vi "七段数码管788.vi"() -> ()   [LabVIEW 2025]
uses:
  <vilib>/Instr/_visa.llb/VISA Configure Serial Port (Instr).vi
panel:
  out "Number of Bytes":u32
  in  "?":bool
  in  "?":bool
  in  "?":bool
  in  "停止":bool
  out "比赛次数个位":T1={"1"=TRUE, "2"=TRUE, "3"=TRUE, "4"=TRUE, "5"=TRUE, "6"=TRUE, "7"=FALSE}
  out "比赛次数十位":T1={"1"=TRUE, "2"=TRUE, "3"=TRUE, "4"=TRUE, "5"=TRUE, "6"=TRUE, "7"=FALSE}
  out "读取缓冲区 5":string
  in  "VISA resource":refnum<visa-resource-name> caption="VISA资源名称"
  out "7 3":bool
  out "6 3":bool
  out "5 3":bool
  out "4 3":bool
  out "3 3":bool
  out "2 3":bool
  out "1 3":bool
  out "7 2":bool
  out "6 2":bool
  out "5 2":bool
  out "4 2":bool
  out "3 2":bool
  out "2 2":bool
  out "1 2":bool
  out "7":bool
  out "6":bool
  out "5":bool
  out "4":bool
  out "3":bool
  out "2":bool
  out "1":bool
  out "结束":bool
  out "计时":bool=TRUE
  out "候场/暂停":bool
  in  "比赛状态":bool
  out "指示灯1 2":bool=TRUE
  out "指示灯2 2":bool=TRUE
  out "蓝方本局得分个位":T1={"1"=TRUE, "2"=TRUE, "3"=TRUE, "4"=TRUE, "5"=TRUE, "6"=TRUE, "7"=FALSE}
  out "蓝方本局得分十位":T1={"1"=TRUE, "2"=TRUE, "3"=TRUE, "4"=TRUE, "5"=TRUE, "6"=TRUE, "7"=FALSE}
  out "红方本局得分个位":T1={"1"=TRUE, "2"=TRUE, "3"=TRUE, "4"=TRUE, "5"=TRUE, "6"=TRUE, "7"=FALSE}
  out "红方本局得分十位":T1={"1"=TRUE, "2"=TRUE, "3"=TRUE, "4"=TRUE, "5"=TRUE, "6"=TRUE, "7"=FALSE}
  out "指示灯2":bool=TRUE
  out "指示灯1":bool=TRUE
  out "蓝方胜场得分个位":T1={"1"=TRUE, "2"=TRUE, "3"=TRUE, "4"=TRUE, "5"=TRUE, "6"=TRUE, "7"=FALSE}
  out "蓝方胜场比分十位":T1={"1"=TRUE, "2"=TRUE, "3"=TRUE, "4"=TRUE, "5"=TRUE, "6"=TRUE, "7"=FALSE}
  out "红方胜场比分个位":T1={"1"=TRUE, "2"=TRUE, "3"=TRUE, "4"=TRUE, "5"=TRUE, "6"=TRUE, "7"=FALSE}
  out "红方胜场比分十位":T1={"1"=TRUE, "2"=TRUE, "3"=TRUE, "4"=TRUE, "5"=TRUE, "6"=TRUE, "7"=FALSE}
  # "竹节人大作战数字擂台"
  # "比赛场次"
  # "比赛倒计时"
  # "红方"
  # "蓝方"
  # "本局得分"
  # "串口配置与操作区"
  # "胜场大比分"
  # "比赛状态"
  # "候场/暂停"
  # "计时"
  # "结束"
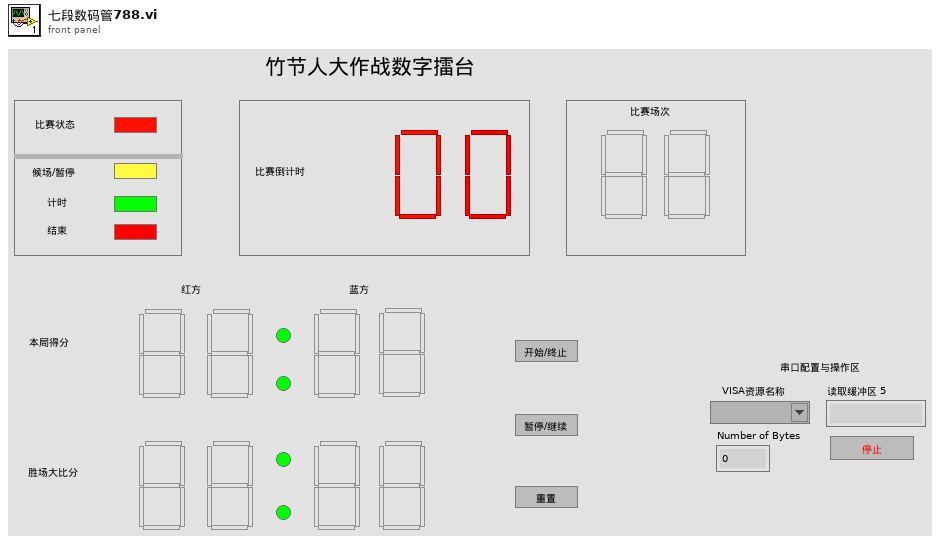
[diagram p1: front panel]
types:
  T1 = cluster{"1":bool, "2":bool, "3":bool, "4":bool, "5":bool, "6":bool, "7":bool}
  T2 = cluster{"7":bool, "6":bool, "5":bool, "4":bool, "3":bool, "2":bool, "1":bool}
  T3 = enum16{"big-endian, network order", "native, host order", "little-endian"}
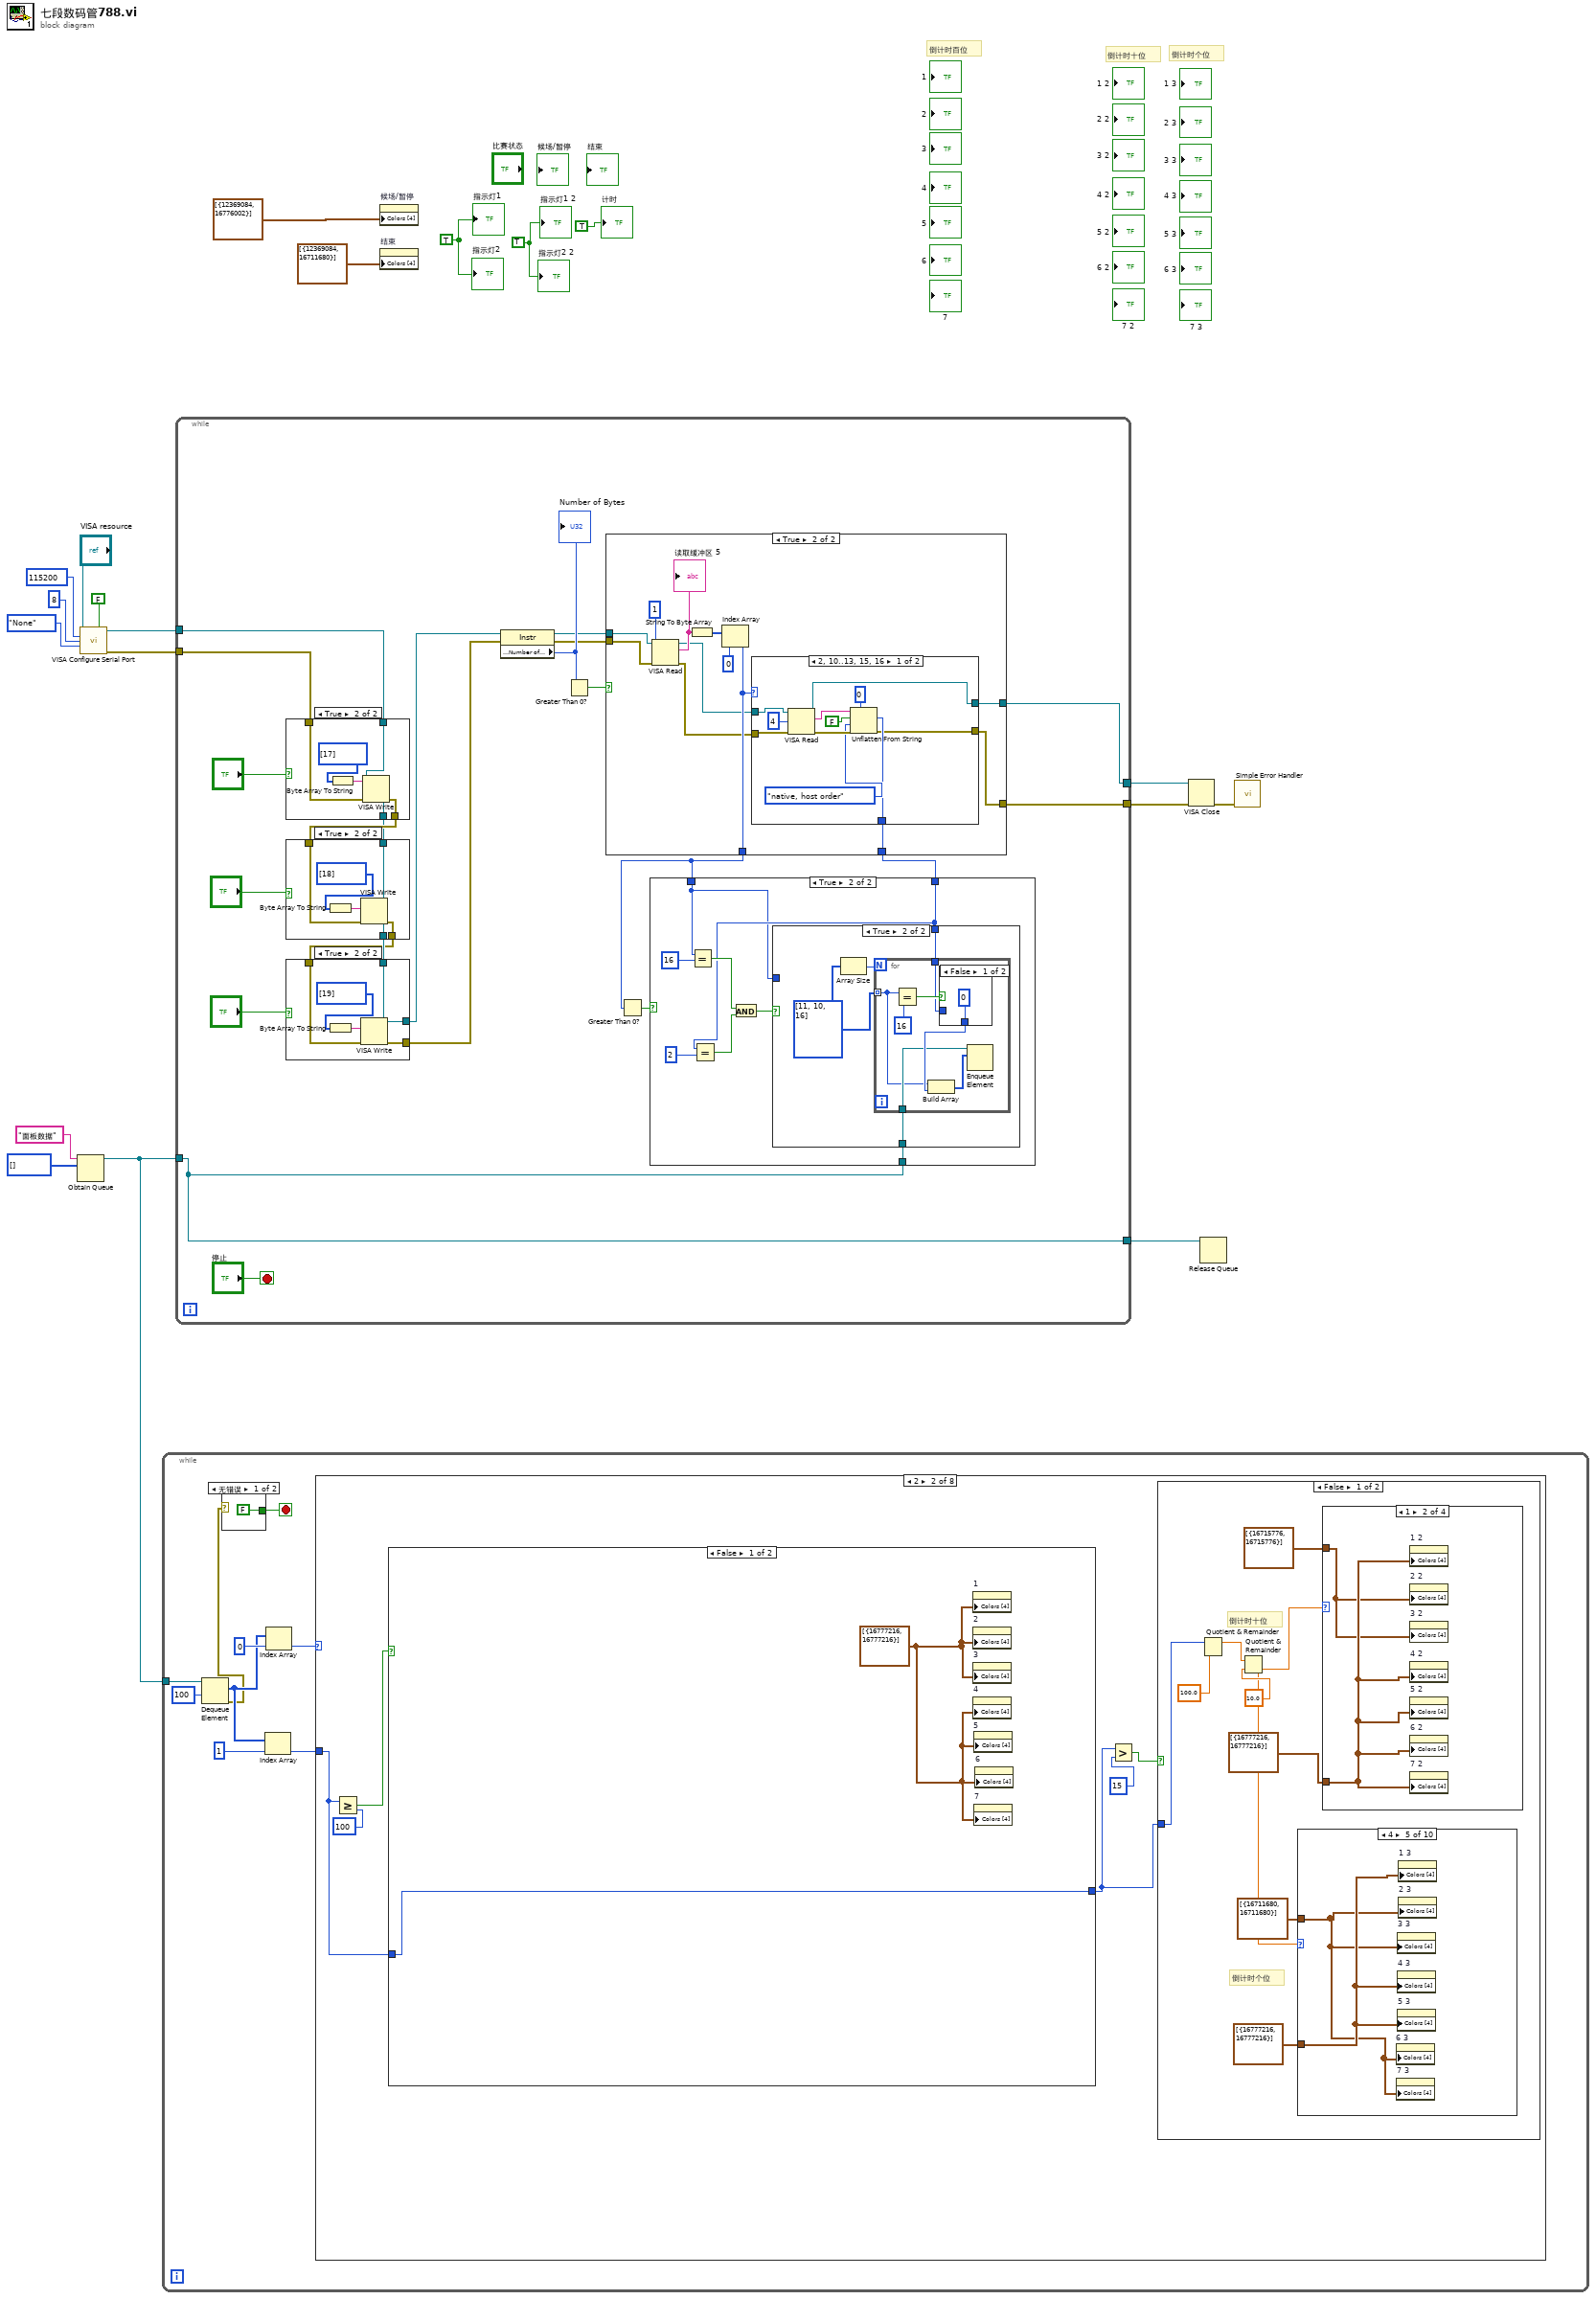
[diagram p0: block diagram]
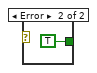
[diagram p2: hidden frame]
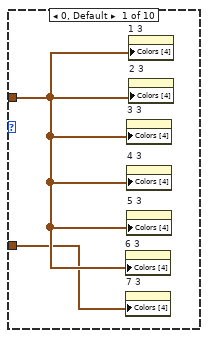
[diagram p4: hidden frame]
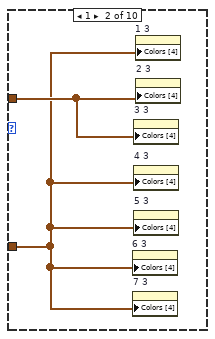
[diagram p5: hidden frame]
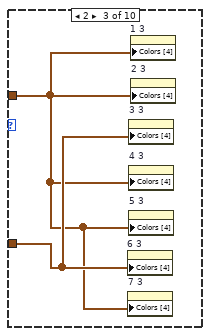
[diagram p6: hidden frame]
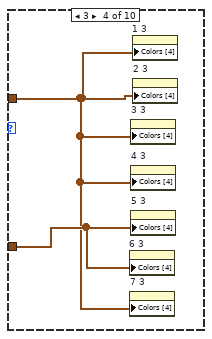
[diagram p7: hidden frame]
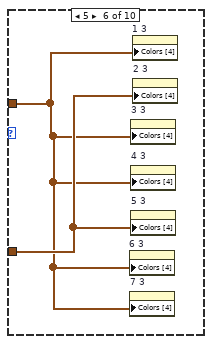
[diagram p8: hidden frame]
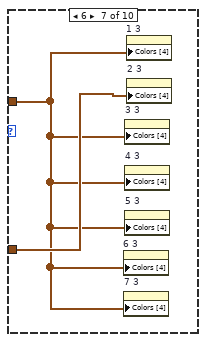
[diagram p9: hidden frame]
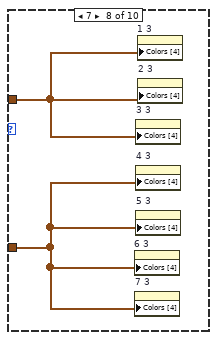
[diagram p10: hidden frame]
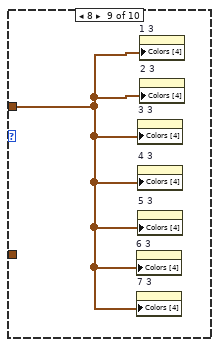
[diagram p11: hidden frame]
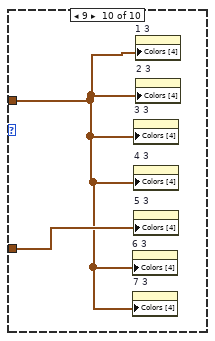
[diagram p12: hidden frame]
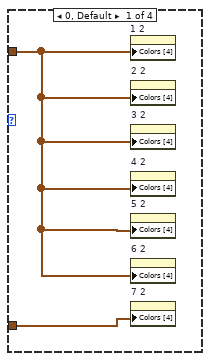
[diagram p13: hidden frame]
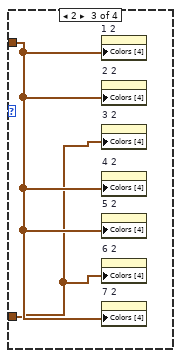
[diagram p14: hidden frame]
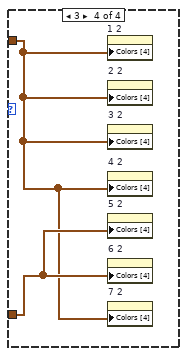
[diagram p15: hidden frame]
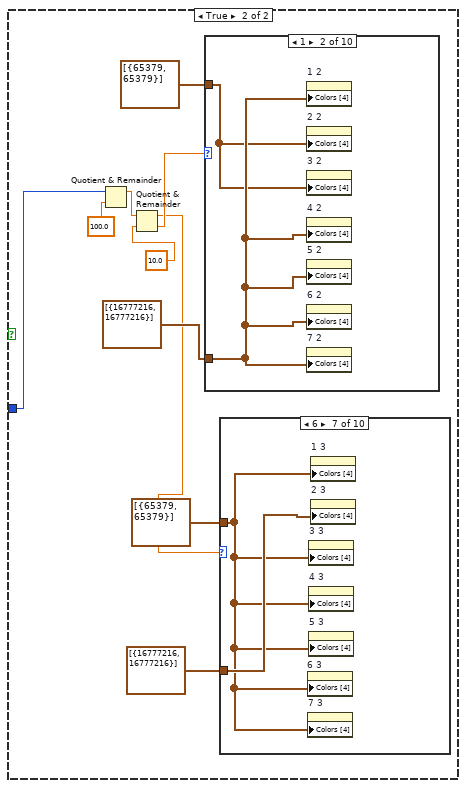
[diagram p16: hidden frame]
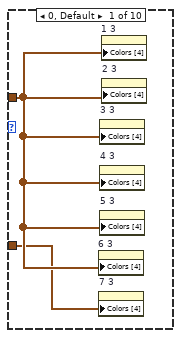
[diagram p17: hidden frame]
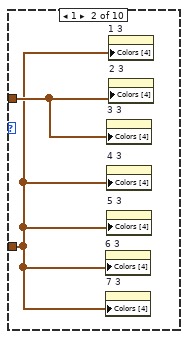
[diagram p18: hidden frame]
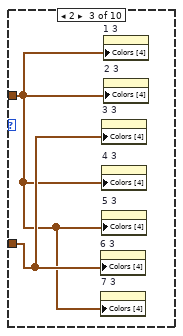
[diagram p19: hidden frame]
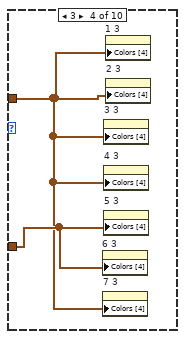
[diagram p20: hidden frame]
diagram:
  w15 = TRUE
  w16 = TRUE
  # "倒计时个位"
  # "倒计时十位"
  # "倒计时百位"
  n1 = Obtain Queue(name (unnamed)="面板数据" ("名称（未命名）"), element data type=i32[] []) -> (queue out=w2:refnum<queue>)  [unwired: 3 in, 2 out]
  n2 = call-poly "VISA Configure Serial Port"("VISA resource name"="VISA resource", "Enable Termination\nChar (T)"=FALSE ("Enable Termination\nChar (T)"), "baud rate (9600)"=u32 115200, "data bits (8)"=u16 8, "parity (0:none)"=enum16{"None", "Odd", "Even", "Mark", "Space"}."None") -> ("VISA resource name out"=w6:refnum<visa-resource-name>, "error out"=w5:errorcluster)  [unwired: 9 in]
  n3 = while {
    tunnel: w2 -> [w23]
    stop <- w24 stop-if-true
    n4 = Dequeue Element(queue=w23, timeout in ms (-1)=100 ("超时毫秒(-1)")) -> (element=w22:i32[], error out=w21:errorcluster)  [unwired: 1 in, 2 out]
    n5 = case shown="无错误" w21 {
      tunnel: [FALSE TRUE] -> w24
      frame No Error {
      }
      frame Error {
      }
    }
    n6 = Index Array(array=w22, index=1 ("索引")) -> (element=w25:i32)
    n7 = Index Array(array=w22, index=0 ("索引")) -> (element=w26:i32)
    n8 = case shown="2" w26 {
      tunnel: w25 -> [_ w33 w190 w219 w246 w271 w297 w321]
      frame Default {
      }
      frame 2 {
        n9 = Greater Or Equal?(x=w33, y=100) -> (x >= y?=w32:bool)
        n10 = case shown="False" w32 {
          tunnel: w33 -> [w123 w124]
          tunnel: [w123 w124] -> w31
          frame False {
            w122 = cluster{u32, u32}[] [{16777216, 16777216}] ("颜色[4]")
            n11 = property on="1" class="Bool (严格)"("Colors [4]"=w122) -> ()  [unwired: 2 in, 2 out]
            n12 = property on="2" class="Bool (严格)"("Colors [4]"=w122) -> ()  [unwired: 2 in, 2 out]
            n13 = property on="3" class="Bool (严格)"("Colors [4]"=w122) -> ()  [unwired: 2 in, 2 out]
            n14 = property on="4" class="Bool (严格)"("Colors [4]"=w122) -> ()  [unwired: 2 in, 2 out]
            n15 = property on="5" class="Bool (严格)"("Colors [4]"=w122) -> ()  [unwired: 2 in, 2 out]
            n16 = property on="7" class="Bool (严格)"("Colors [4]"=w122) -> ()  [unwired: 2 in, 2 out]
            n17 = property on="6" class="Bool (严格)"("Colors [4]"=w122) -> ()  [unwired: 2 in, 2 out]
          }
          frame True {
            w125 = cluster{u32, u32}[] [{16777216, 16777216}] ("颜色[4]")
            w126 = cluster{u32, u32}[] [{65379, 65379}] ("颜色[4]")
            n18 = Quotient & Remainder(x=w124, y=100.0) -> (x-y*floor(x/y)=w132:dbl, floor(x/y)=w128:dbl)
            n19 = Quotient & Remainder(x=w132, y=10.0) -> (x-y*floor(x/y)=w130:dbl, floor(x/y)=w131:dbl)
            n20 = case shown="0, 默认" w128 {
              tunnel: w126 -> [w172 w174 w176 w178 w180 w182 w184 w186 w187 w189]
              tunnel: w125 -> [w171 w173 w175 w177 w179 w181 w183 w185 _ w188]
              frame 0, Default {
                n21 = property on="1" class="Bool (严格)"("Colors [4]"=w172) -> ()  [unwired: 2 in, 2 out]
                n22 = property on="2" class="Bool (严格)"("Colors [4]"=w172) -> ()  [unwired: 2 in, 2 out]
                n23 = property on="5" class="Bool (严格)"("Colors [4]"=w172) -> ()  [unwired: 2 in, 2 out]
                n24 = property on="3" class="Bool (严格)"("Colors [4]"=w172) -> ()  [unwired: 2 in, 2 out]
                n25 = property on="4" class="Bool (严格)"("Colors [4]"=w172) -> ()  [unwired: 2 in, 2 out]
                n26 = property on="7" class="Bool (严格)"("Colors [4]"=w171) -> ()  [unwired: 2 in, 2 out]
                n27 = property on="6" class="Bool (严格)"("Colors [4]"=w172) -> ()  [unwired: 2 in, 2 out]
              }
              frame 1 {
                n28 = property on="1" class="Bool (严格)"("Colors [4]"=w173) -> ()  [unwired: 2 in, 2 out]
                n29 = property on="2" class="Bool (严格)"("Colors [4]"=w174) -> ()  [unwired: 2 in, 2 out]
                n30 = property on="5" class="Bool (严格)"("Colors [4]"=w173) -> ()  [unwired: 2 in, 2 out]
                n31 = property on="3" class="Bool (严格)"("Colors [4]"=w174) -> ()  [unwired: 2 in, 2 out]
                n32 = property on="4" class="Bool (严格)"("Colors [4]"=w173) -> ()  [unwired: 2 in, 2 out]
                n33 = property on="7" class="Bool (严格)"("Colors [4]"=w173) -> ()  [unwired: 2 in, 2 out]
                n34 = property on="6" class="Bool (严格)"("Colors [4]"=w173) -> ()  [unwired: 2 in, 2 out]
              }
              frame 2 {
                n35 = property on="1" class="Bool (严格)"("Colors [4]"=w176) -> ()  [unwired: 2 in, 2 out]
                n36 = property on="2" class="Bool (严格)"("Colors [4]"=w176) -> ()  [unwired: 2 in, 2 out]
                n37 = property on="3" class="Bool (严格)"("Colors [4]"=w175) -> ()  [unwired: 2 in, 2 out]
                n38 = property on="4" class="Bool (严格)"("Colors [4]"=w176) -> ()  [unwired: 2 in, 2 out]
                n39 = property on="5" class="Bool (严格)"("Colors [4]"=w176) -> ()  [unwired: 2 in, 2 out]
                n40 = property on="7" class="Bool (严格)"("Colors [4]"=w176) -> ()  [unwired: 2 in, 2 out]
                n41 = property on="6" class="Bool (严格)"("Colors [4]"=w175) -> ()  [unwired: 2 in, 2 out]
              }
              frame 3 {
                n42 = property on="1" class="Bool (严格)"("Colors [4]"=w178) -> ()  [unwired: 2 in, 2 out]
                n43 = property on="2" class="Bool (严格)"("Colors [4]"=w178) -> ()  [unwired: 2 in, 2 out]
                n44 = property on="3" class="Bool (严格)"("Colors [4]"=w178) -> ()  [unwired: 2 in, 2 out]
                n45 = property on="4" class="Bool (严格)"("Colors [4]"=w178) -> ()  [unwired: 2 in, 2 out]
                n46 = property on="5" class="Bool (严格)"("Colors [4]"=w177) -> ()  [unwired: 2 in, 2 out]
                n47 = property on="7" class="Bool (严格)"("Colors [4]"=w178) -> ()  [unwired: 2 in, 2 out]
                n48 = property on="6" class="Bool (严格)"("Colors [4]"=w177) -> ()  [unwired: 2 in, 2 out]
              }
              frame 4 {
                n49 = property on="1" class="Bool (严格)"("Colors [4]"=w179) -> ()  [unwired: 2 in, 2 out]
                n50 = property on="2" class="Bool (严格)"("Colors [4]"=w180) -> ()  [unwired: 2 in, 2 out]
                n51 = property on="3" class="Bool (严格)"("Colors [4]"=w180) -> ()  [unwired: 2 in, 2 out]
                n52 = property on="4" class="Bool (严格)"("Colors [4]"=w179) -> ()  [unwired: 2 in, 2 out]
                n53 = property on="5" class="Bool (严格)"("Colors [4]"=w179) -> ()  [unwired: 2 in, 2 out]
                n54 = property on="7" class="Bool (严格)"("Colors [4]"=w180) -> ()  [unwired: 2 in, 2 out]
                n55 = property on="6" class="Bool (严格)"("Colors [4]"=w180) -> ()  [unwired: 2 in, 2 out]
              }
              frame 5 {
                n56 = property on="1" class="Bool (严格)"("Colors [4]"=w182) -> ()  [unwired: 2 in, 2 out]
                n57 = property on="2" class="Bool (严格)"("Colors [4]"=w181) -> ()  [unwired: 2 in, 2 out]
                n58 = property on="3" class="Bool (严格)"("Colors [4]"=w182) -> ()  [unwired: 2 in, 2 out]
                n59 = property on="4" class="Bool (严格)"("Colors [4]"=w182) -> ()  [unwired: 2 in, 2 out]
                n60 = property on="5" class="Bool (严格)"("Colors [4]"=w181) -> ()  [unwired: 2 in, 2 out]
                n61 = property on="7" class="Bool (严格)"("Colors [4]"=w182) -> ()  [unwired: 2 in, 2 out]
                n62 = property on="6" class="Bool (严格)"("Colors [4]"=w182) -> ()  [unwired: 2 in, 2 out]
              }
              frame 6 {
                n63 = property on="1" class="Bool (严格)"("Colors [4]"=w184) -> ()  [unwired: 2 in, 2 out]
                n64 = property on="2" class="Bool (严格)"("Colors [4]"=w183) -> ()  [unwired: 2 in, 2 out]
                n65 = property on="3" class="Bool (严格)"("Colors [4]"=w184) -> ()  [unwired: 2 in, 2 out]
                n66 = property on="4" class="Bool (严格)"("Colors [4]"=w184) -> ()  [unwired: 2 in, 2 out]
                n67 = property on="5" class="Bool (严格)"("Colors [4]"=w184) -> ()  [unwired: 2 in, 2 out]
                n68 = property on="7" class="Bool (严格)"("Colors [4]"=w184) -> ()  [unwired: 2 in, 2 out]
                n69 = property on="6" class="Bool (严格)"("Colors [4]"=w184) -> ()  [unwired: 2 in, 2 out]
              }
              frame 7 {
                n70 = property on="1" class="Bool (严格)"("Colors [4]"=w186) -> ()  [unwired: 2 in, 2 out]
                n71 = property on="2" class="Bool (严格)"("Colors [4]"=w186) -> ()  [unwired: 2 in, 2 out]
                n72 = property on="3" class="Bool (严格)"("Colors [4]"=w186) -> ()  [unwired: 2 in, 2 out]
                n73 = property on="4" class="Bool (严格)"("Colors [4]"=w185) -> ()  [unwired: 2 in, 2 out]
                n74 = property on="5" class="Bool (严格)"("Colors [4]"=w185) -> ()  [unwired: 2 in, 2 out]
                n75 = property on="7" class="Bool (严格)"("Colors [4]"=w185) -> ()  [unwired: 2 in, 2 out]
                n76 = property on="6" class="Bool (严格)"("Colors [4]"=w185) -> ()  [unwired: 2 in, 2 out]
              }
              frame 8 {
                n77 = property on="1" class="Bool (严格)"("Colors [4]"=w187) -> ()  [unwired: 2 in, 2 out]
                n78 = property on="2" class="Bool (严格)"("Colors [4]"=w187) -> ()  [unwired: 2 in, 2 out]
                n79 = property on="3" class="Bool (严格)"("Colors [4]"=w187) -> ()  [unwired: 2 in, 2 out]
                n80 = property on="4" class="Bool (严格)"("Colors [4]"=w187) -> ()  [unwired: 2 in, 2 out]
                n81 = property on="5" class="Bool (严格)"("Colors [4]"=w187) -> ()  [unwired: 2 in, 2 out]
                n82 = property on="7" class="Bool (严格)"("Colors [4]"=w187) -> ()  [unwired: 2 in, 2 out]
                n83 = property on="6" class="Bool (严格)"("Colors [4]"=w187) -> ()  [unwired: 2 in, 2 out]
              }
              frame 9 {
                n84 = property on="1" class="Bool (严格)"("Colors [4]"=w189) -> ()  [unwired: 2 in, 2 out]
                n85 = property on="2" class="Bool (严格)"("Colors [4]"=w189) -> ()  [unwired: 2 in, 2 out]
                n86 = property on="3" class="Bool (严格)"("Colors [4]"=w189) -> ()  [unwired: 2 in, 2 out]
                n87 = property on="4" class="Bool (严格)"("Colors [4]"=w189) -> ()  [unwired: 2 in, 2 out]
                n88 = property on="5" class="Bool (严格)"("Colors [4]"=w188) -> ()  [unwired: 2 in, 2 out]
                n89 = property on="7" class="Bool (严格)"("Colors [4]"=w189) -> ()  [unwired: 2 in, 2 out]
                n90 = property on="6" class="Bool (严格)"("Colors [4]"=w189) -> ()  [unwired: 2 in, 2 out]
              }
            }
            n91 = case shown="0, 默认" w130 {
              tunnel: w126 -> [w134 w136 w137 w139 w141 w143 w145 w148 w149 w150]
              tunnel: w125 -> [w133 w135 w138 w140 w142 w144 w146 w147 _ w151]
              frame 0, Default {
                n92 = property on="6 3" class="Bool (严格)"("Colors [4]"=w134) -> ()  [unwired: 2 in, 2 out]
                n93 = property on="7 3" class="Bool (严格)"("Colors [4]"=w133) -> ()  [unwired: 2 in, 2 out]
                n94 = property on="3 3" class="Bool (严格)"("Colors [4]"=w134) -> ()  [unwired: 2 in, 2 out]
                n95 = property on="4 3" class="Bool (严格)"("Colors [4]"=w134) -> ()  [unwired: 2 in, 2 out]
                n96 = property on="5 3" class="Bool (严格)"("Colors [4]"=w134) -> ()  [unwired: 2 in, 2 out]
                n97 = property on="1 3" class="Bool (严格)"("Colors [4]"=w134) -> ()  [unwired: 2 in, 2 out]
                n98 = property on="2 3" class="Bool (严格)"("Colors [4]"=w134) -> ()  [unwired: 2 in, 2 out]
              }
              frame 1 {
                n99 = property on="6 3" class="Bool (严格)"("Colors [4]"=w135) -> ()  [unwired: 2 in, 2 out]
                n100 = property on="7 3" class="Bool (严格)"("Colors [4]"=w135) -> ()  [unwired: 2 in, 2 out]
                n101 = property on="3 3" class="Bool (严格)"("Colors [4]"=w136) -> ()  [unwired: 2 in, 2 out]
                n102 = property on="4 3" class="Bool (严格)"("Colors [4]"=w135) -> ()  [unwired: 2 in, 2 out]
                n103 = property on="5 3" class="Bool (严格)"("Colors [4]"=w135) -> ()  [unwired: 2 in, 2 out]
                n104 = property on="1 3" class="Bool (严格)"("Colors [4]"=w135) -> ()  [unwired: 2 in, 2 out]
                n105 = property on="2 3" class="Bool (严格)"("Colors [4]"=w136) -> ()  [unwired: 2 in, 2 out]
              }
              frame 2 {
                n106 = property on="6 3" class="Bool (严格)"("Colors [4]"=w138) -> ()  [unwired: 2 in, 2 out]
                n107 = property on="7 3" class="Bool (严格)"("Colors [4]"=w137) -> ()  [unwired: 2 in, 2 out]
                n108 = property on="3 3" class="Bool (严格)"("Colors [4]"=w138) -> ()  [unwired: 2 in, 2 out]
                n109 = property on="4 3" class="Bool (严格)"("Colors [4]"=w137) -> ()  [unwired: 2 in, 2 out]
                n110 = property on="5 3" class="Bool (严格)"("Colors [4]"=w137) -> ()  [unwired: 2 in, 2 out]
                n111 = property on="1 3" class="Bool (严格)"("Colors [4]"=w137) -> ()  [unwired: 2 in, 2 out]
                n112 = property on="2 3" class="Bool (严格)"("Colors [4]"=w137) -> ()  [unwired: 2 in, 2 out]
              }
              frame 3 {
                n113 = property on="6 3" class="Bool (严格)"("Colors [4]"=w140) -> ()  [unwired: 2 in, 2 out]
                n114 = property on="7 3" class="Bool (严格)"("Colors [4]"=w139) -> ()  [unwired: 2 in, 2 out]
                n115 = property on="3 3" class="Bool (严格)"("Colors [4]"=w139) -> ()  [unwired: 2 in, 2 out]
                n116 = property on="4 3" class="Bool (严格)"("Colors [4]"=w139) -> ()  [unwired: 2 in, 2 out]
                n117 = property on="5 3" class="Bool (严格)"("Colors [4]"=w140) -> ()  [unwired: 2 in, 2 out]
                n118 = property on="1 3" class="Bool (严格)"("Colors [4]"=w139) -> ()  [unwired: 2 in, 2 out]
                n119 = property on="2 3" class="Bool (严格)"("Colors [4]"=w139) -> ()  [unwired: 2 in, 2 out]
              }
              frame 4 {
                n120 = property on="6 3" class="Bool (严格)"("Colors [4]"=w141) -> ()  [unwired: 2 in, 2 out]
                n121 = property on="7 3" class="Bool (严格)"("Colors [4]"=w141) -> ()  [unwired: 2 in, 2 out]
                n122 = property on="3 3" class="Bool (严格)"("Colors [4]"=w141) -> ()  [unwired: 2 in, 2 out]
                n123 = property on="4 3" class="Bool (严格)"("Colors [4]"=w142) -> ()  [unwired: 2 in, 2 out]
                n124 = property on="5 3" class="Bool (严格)"("Colors [4]"=w142) -> ()  [unwired: 2 in, 2 out]
                n125 = property on="1 3" class="Bool (严格)"("Colors [4]"=w142) -> ()  [unwired: 2 in, 2 out]
                n126 = property on="2 3" class="Bool (严格)"("Colors [4]"=w141) -> ()  [unwired: 2 in, 2 out]
              }
              frame 5 {
                n127 = property on="6 3" class="Bool (严格)"("Colors [4]"=w143) -> ()  [unwired: 2 in, 2 out]
                n128 = property on="7 3" class="Bool (严格)"("Colors [4]"=w143) -> ()  [unwired: 2 in, 2 out]
                n129 = property on="3 3" class="Bool (严格)"("Colors [4]"=w143) -> ()  [unwired: 2 in, 2 out]
                n130 = property on="4 3" class="Bool (严格)"("Colors [4]"=w143) -> ()  [unwired: 2 in, 2 out]
                n131 = property on="5 3" class="Bool (严格)"("Colors [4]"=w144) -> ()  [unwired: 2 in, 2 out]
                n132 = property on="1 3" class="Bool (严格)"("Colors [4]"=w143) -> ()  [unwired: 2 in, 2 out]
                n133 = property on="2 3" class="Bool (严格)"("Colors [4]"=w144) -> ()  [unwired: 2 in, 2 out]
              }
              frame 6 {
                n134 = property on="6 3" class="Bool (严格)"("Colors [4]"=w145) -> ()  [unwired: 2 in, 2 out]
                n135 = property on="7 3" class="Bool (严格)"("Colors [4]"=w145) -> ()  [unwired: 2 in, 2 out]
                n136 = property on="3 3" class="Bool (严格)"("Colors [4]"=w145) -> ()  [unwired: 2 in, 2 out]
                n137 = property on="4 3" class="Bool (严格)"("Colors [4]"=w145) -> ()  [unwired: 2 in, 2 out]
                n138 = property on="5 3" class="Bool (严格)"("Colors [4]"=w145) -> ()  [unwired: 2 in, 2 out]
                n139 = property on="1 3" class="Bool (严格)"("Colors [4]"=w145) -> ()  [unwired: 2 in, 2 out]
                n140 = property on="2 3" class="Bool (严格)"("Colors [4]"=w146) -> ()  [unwired: 2 in, 2 out]
              }
              frame 7 {
                n141 = property on="6 3" class="Bool (严格)"("Colors [4]"=w147) -> ()  [unwired: 2 in, 2 out]
                n142 = property on="7 3" class="Bool (严格)"("Colors [4]"=w147) -> ()  [unwired: 2 in, 2 out]
                n143 = property on="3 3" class="Bool (严格)"("Colors [4]"=w148) -> ()  [unwired: 2 in, 2 out]
                n144 = property on="4 3" class="Bool (严格)"("Colors [4]"=w147) -> ()  [unwired: 2 in, 2 out]
                n145 = property on="5 3" class="Bool (严格)"("Colors [4]"=w147) -> ()  [unwired: 2 in, 2 out]
                n146 = property on="1 3" class="Bool (严格)"("Colors [4]"=w148) -> ()  [unwired: 2 in, 2 out]
                n147 = property on="2 3" class="Bool (严格)"("Colors [4]"=w148) -> ()  [unwired: 2 in, 2 out]
              }
              frame 8 {
                n148 = property on="6 3" class="Bool (严格)"("Colors [4]"=w149) -> ()  [unwired: 2 in, 2 out]
                n149 = property on="7 3" class="Bool (严格)"("Colors [4]"=w149) -> ()  [unwired: 2 in, 2 out]
                n150 = property on="3 3" class="Bool (严格)"("Colors [4]"=w149) -> ()  [unwired: 2 in, 2 out]
                n151 = property on="4 3" class="Bool (严格)"("Colors [4]"=w149) -> ()  [unwired: 2 in, 2 out]
                n152 = property on="5 3" class="Bool (严格)"("Colors [4]"=w149) -> ()  [unwired: 2 in, 2 out]
                n153 = property on="1 3" class="Bool (严格)"("Colors [4]"=w149) -> ()  [unwired: 2 in, 2 out]
                n154 = property on="2 3" class="Bool (严格)"("Colors [4]"=w149) -> ()  [unwired: 2 in, 2 out]
              }
              frame 9 {
                n155 = property on="6 3" class="Bool (严格)"("Colors [4]"=w150) -> ()  [unwired: 2 in, 2 out]
                n156 = property on="7 3" class="Bool (严格)"("Colors [4]"=w150) -> ()  [unwired: 2 in, 2 out]
                n157 = property on="3 3" class="Bool (严格)"("Colors [4]"=w150) -> ()  [unwired: 2 in, 2 out]
                n158 = property on="4 3" class="Bool (严格)"("Colors [4]"=w150) -> ()  [unwired: 2 in, 2 out]
                n159 = property on="5 3" class="Bool (严格)"("Colors [4]"=w151) -> ()  [unwired: 2 in, 2 out]
                n160 = property on="1 3" class="Bool (严格)"("Colors [4]"=w150) -> ()  [unwired: 2 in, 2 out]
                n161 = property on="2 3" class="Bool (严格)"("Colors [4]"=w150) -> ()  [unwired: 2 in, 2 out]
              }
            }
            n162 = case shown="0, 默认" w131 {
              tunnel: w126 -> [w153 w154 w157 w158 w160 w162 w164 w167 w168 w169]
              tunnel: w125 -> [w152 w155 w156 w159 w161 w163 w165 w166 _ w170]
              frame 0, Default {
                n163 = property on="1 2" class="Bool (严格)"("Colors [4]"=w153) -> ()  [unwired: 2 in, 2 out]
                n164 = property on="2 2" class="Bool (严格)"("Colors [4]"=w153) -> ()  [unwired: 2 in, 2 out]
                n165 = property on="3 2" class="Bool (严格)"("Colors [4]"=w153) -> ()  [unwired: 2 in, 2 out]
                n166 = property on="4 2" class="Bool (严格)"("Colors [4]"=w153) -> ()  [unwired: 2 in, 2 out]
                n167 = property on="5 2" class="Bool (严格)"("Colors [4]"=w153) -> ()  [unwired: 2 in, 2 out]
                n168 = property on="6 2" class="Bool (严格)"("Colors [4]"=w153) -> ()  [unwired: 2 in, 2 out]
                n169 = property on="7 2" class="Bool (严格)"("Colors [4]"=w152) -> ()  [unwired: 2 in, 2 out]
              }
              frame 1 {
                n170 = property on="1 2" class="Bool (严格)"("Colors [4]"=w155) -> ()  [unwired: 2 in, 2 out]
                n171 = property on="2 2" class="Bool (严格)"("Colors [4]"=w154) -> ()  [unwired: 2 in, 2 out]
                n172 = property on="3 2" class="Bool (严格)"("Colors [4]"=w154) -> ()  [unwired: 2 in, 2 out]
                n173 = property on="4 2" class="Bool (严格)"("Colors [4]"=w155) -> ()  [unwired: 2 in, 2 out]
                n174 = property on="5 2" class="Bool (严格)"("Colors [4]"=w155) -> ()  [unwired: 2 in, 2 out]
                n175 = property on="6 2" class="Bool (严格)"("Colors [4]"=w155) -> ()  [unwired: 2 in, 2 out]
                n176 = property on="7 2" class="Bool (严格)"("Colors [4]"=w155) -> ()  [unwired: 2 in, 2 out]
              }
              frame 2 {
                n177 = property on="1 2" class="Bool (严格)"("Colors [4]"=w157) -> ()  [unwired: 2 in, 2 out]
                n178 = property on="2 2" class="Bool (严格)"("Colors [4]"=w157) -> ()  [unwired: 2 in, 2 out]
                n179 = property on="3 2" class="Bool (严格)"("Colors [4]"=w156) -> ()  [unwired: 2 in, 2 out]
                n180 = property on="4 2" class="Bool (严格)"("Colors [4]"=w157) -> ()  [unwired: 2 in, 2 out]
                n181 = property on="5 2" class="Bool (严格)"("Colors [4]"=w157) -> ()  [unwired: 2 in, 2 out]
                n182 = property on="6 2" class="Bool (严格)"("Colors [4]"=w156) -> ()  [unwired: 2 in, 2 out]
                n183 = property on="7 2" class="Bool (严格)"("Colors [4]"=w157) -> ()  [unwired: 2 in, 2 out]
              }
              frame 3 {
                n184 = property on="1 2" class="Bool (严格)"("Colors [4]"=w158) -> ()  [unwired: 2 in, 2 out]
                n185 = property on="2 2" class="Bool (严格)"("Colors [4]"=w158) -> ()  [unwired: 2 in, 2 out]
                n186 = property on="3 2" class="Bool (严格)"("Colors [4]"=w158) -> ()  [unwired: 2 in, 2 out]
                n187 = property on="4 2" class="Bool (严格)"("Colors [4]"=w158) -> ()  [unwired: 2 in, 2 out]
                n188 = property on="5 2" class="Bool (严格)"("Colors [4]"=w159) -> ()  [unwired: 2 in, 2 out]
                n189 = property on="6 2" class="Bool (严格)"("Colors [4]"=w159) -> ()  [unwired: 2 in, 2 out]
                n190 = property on="7 2" class="Bool (严格)"("Colors [4]"=w158) -> ()  [unwired: 2 in, 2 out]
              }
              frame 4 {
                n191 = property on="1 2" class="Bool (严格)"("Colors [4]"=w161) -> ()  [unwired: 2 in, 2 out]
                n192 = property on="2 2" class="Bool (严格)"("Colors [4]"=w160) -> ()  [unwired: 2 in, 2 out]
                n193 = property on="3 2" class="Bool (严格)"("Colors [4]"=w160) -> ()  [unwired: 2 in, 2 out]
                n194 = property on="4 2" class="Bool (严格)"("Colors [4]"=w161) -> ()  [unwired: 2 in, 2 out]
                n195 = property on="5 2" class="Bool (严格)"("Colors [4]"=w161) -> ()  [unwired: 2 in, 2 out]
                n196 = property on="6 2" class="Bool (严格)"("Colors [4]"=w160) -> ()  [unwired: 2 in, 2 out]
                n197 = property on="7 2" class="Bool (严格)"("Colors [4]"=w160) -> ()  [unwired: 2 in, 2 out]
              }
              frame 5 {
                n198 = property on="1 2" class="Bool (严格)"("Colors [4]"=w162) -> ()  [unwired: 2 in, 2 out]
                n199 = property on="2 2" class="Bool (严格)"("Colors [4]"=w163) -> ()  [unwired: 2 in, 2 out]
                n200 = property on="3 2" class="Bool (严格)"("Colors [4]"=w162) -> ()  [unwired: 2 in, 2 out]
                n201 = property on="4 2" class="Bool (严格)"("Colors [4]"=w162) -> ()  [unwired: 2 in, 2 out]
                n202 = property on="5 2" class="Bool (严格)"("Colors [4]"=w163) -> ()  [unwired: 2 in, 2 out]
                n203 = property on="6 2" class="Bool (严格)"("Colors [4]"=w162) -> ()  [unwired: 2 in, 2 out]
                n204 = property on="7 2" class="Bool (严格)"("Colors [4]"=w162) -> ()  [unwired: 2 in, 2 out]
              }
              frame 6 {
                n205 = property on="1 2" class="Bool (严格)"("Colors [4]"=w164) -> ()  [unwired: 2 in, 2 out]
                n206 = property on="2 2" class="Bool (严格)"("Colors [4]"=w165) -> ()  [unwired: 2 in, 2 out]
                n207 = property on="3 2" class="Bool (严格)"("Colors [4]"=w164) -> ()  [unwired: 2 in, 2 out]
                n208 = property on="4 2" class="Bool (严格)"("Colors [4]"=w164) -> ()  [unwired: 2 in, 2 out]
                n209 = property on="5 2" class="Bool (严格)"("Colors [4]"=w164) -> ()  [unwired: 2 in, 2 out]
                n210 = property on="6 2" class="Bool (严格)"("Colors [4]"=w164) -> ()  [unwired: 2 in, 2 out]
                n211 = property on="7 2" class="Bool (严格)"("Colors [4]"=w164) -> ()  [unwired: 2 in, 2 out]
              }
              frame 7 {
                n212 = property on="1 2" class="Bool (严格)"("Colors [4]"=w167) -> ()  [unwired: 2 in, 2 out]
                n213 = property on="2 2" class="Bool (严格)"("Colors [4]"=w167) -> ()  [unwired: 2 in, 2 out]
                n214 = property on="3 2" class="Bool (严格)"("Colors [4]"=w167) -> ()  [unwired: 2 in, 2 out]
                n215 = property on="4 2" class="Bool (严格)"("Colors [4]"=w166) -> ()  [unwired: 2 in, 2 out]
                n216 = property on="5 2" class="Bool (严格)"("Colors [4]"=w166) -> ()  [unwired: 2 in, 2 out]
                n217 = property on="6 2" class="Bool (严格)"("Colors [4]"=w166) -> ()  [unwired: 2 in, 2 out]
                n218 = property on="7 2" class="Bool (严格)"("Colors [4]"=w166) -> ()  [unwired: 2 in, 2 out]
              }
              frame 8 {
                n219 = property on="1 2" class="Bool (严格)"("Colors [4]"=w168) -> ()  [unwired: 2 in, 2 out]
                n220 = property on="2 2" class="Bool (严格)"("Colors [4]"=w168) -> ()  [unwired: 2 in, 2 out]
                n221 = property on="3 2" class="Bool (严格)"("Colors [4]"=w168) -> ()  [unwired: 2 in, 2 out]
                n222 = property on="4 2" class="Bool (严格)"("Colors [4]"=w168) -> ()  [unwired: 2 in, 2 out]
                n223 = property on="5 2" class="Bool (严格)"("Colors [4]"=w168) -> ()  [unwired: 2 in, 2 out]
                n224 = property on="6 2" class="Bool (严格)"("Colors [4]"=w168) -> ()  [unwired: 2 in, 2 out]
                n225 = property on="7 2" class="Bool (严格)"("Colors [4]"=w168) -> ()  [unwired: 2 in, 2 out]
              }
              frame 9 {
                n226 = property on="1 2" class="Bool (严格)"("Colors [4]"=w169) -> ()  [unwired: 2 in, 2 out]
                n227 = property on="2 2" class="Bool (严格)"("Colors [4]"=w169) -> ()  [unwired: 2 in, 2 out]
                n228 = property on="3 2" class="Bool (严格)"("Colors [4]"=w169) -> ()  [unwired: 2 in, 2 out]
                n229 = property on="4 2" class="Bool (严格)"("Colors [4]"=w169) -> ()  [unwired: 2 in, 2 out]
                n230 = property on="5 2" class="Bool (严格)"("Colors [4]"=w170) -> ()  [unwired: 2 in, 2 out]
                n231 = property on="6 2" class="Bool (严格)"("Colors [4]"=w169) -> ()  [unwired: 2 in, 2 out]
                n232 = property on="7 2" class="Bool (严格)"("Colors [4]"=w169) -> ()  [unwired: 2 in, 2 out]
              }
            }
          }
        }
        n233 = Greater?(x=w31, y=15) -> (0:w36:bool)
        n234 = case shown="False" w36 {
          tunnel: w31 -> [w38 w77]
          frame False {
            # "倒计时个位"
            # "倒计时十位"
            n235 = Quotient & Remainder(x=w38, y=100.0) -> (x-y*floor(x/y)=w45:dbl)  [unwired: 1 out]
            n236 = Quotient & Remainder(x=w45, y=10.0) -> (x-y*floor(x/y)=w37:dbl, floor(x/y)=w46:dbl)
            n237 = case shown="4" w37 {
              tunnel: cluster{u32, u32}[] [{16711680, 16711680}] ("颜色[4]") -> [w48 w50 w51 w53 w55 w57 w59 w62 w63 w64]
              tunnel: cluster{u32, u32}[] [{16777216, 16777216}] ("颜色[4]") -> [w47 w49 w52 w54 w56 w58 w60 w61 _ w65]
              frame 0, Default {
                n238 = property on="6 3" class="Bool (严格)"("Colors [4]"=w48) -> ()  [unwired: 2 in, 2 out]
                n239 = property on="7 3" class="Bool (严格)"("Colors [4]"=w47) -> ()  [unwired: 2 in, 2 out]
                n240 = property on="3 3" class="Bool (严格)"("Colors [4]"=w48) -> ()  [unwired: 2 in, 2 out]
                n241 = property on="4 3" class="Bool (严格)"("Colors [4]"=w48) -> ()  [unwired: 2 in, 2 out]
                n242 = property on="5 3" class="Bool (严格)"("Colors [4]"=w48) -> ()  [unwired: 2 in, 2 out]
                n243 = property on="1 3" class="Bool (严格)"("Colors [4]"=w48) -> ()  [unwired: 2 in, 2 out]
                n244 = property on="2 3" class="Bool (严格)"("Colors [4]"=w48) -> ()  [unwired: 2 in, 2 out]
              }
              frame 1 {
                n245 = property on="6 3" class="Bool (严格)"("Colors [4]"=w49) -> ()  [unwired: 2 in, 2 out]
                n246 = property on="7 3" class="Bool (严格)"("Colors [4]"=w49) -> ()  [unwired: 2 in, 2 out]
                n247 = property on="3 3" class="Bool (严格)"("Colors [4]"=w50) -> ()  [unwired: 2 in, 2 out]
                n248 = property on="4 3" class="Bool (严格)"("Colors [4]"=w49) -> ()  [unwired: 2 in, 2 out]
                n249 = property on="5 3" class="Bool (严格)"("Colors [4]"=w49) -> ()  [unwired: 2 in, 2 out]
                n250 = property on="1 3" class="Bool (严格)"("Colors [4]"=w49) -> ()  [unwired: 2 in, 2 out]
                n251 = property on="2 3" class="Bool (严格)"("Colors [4]"=w50) -> ()  [unwired: 2 in, 2 out]
              }
              frame 2 {
                n252 = property on="6 3" class="Bool (严格)"("Colors [4]"=w52) -> ()  [unwired: 2 in, 2 out]
                n253 = property on="7 3" class="Bool (严格)"("Colors [4]"=w51) -> ()  [unwired: 2 in, 2 out]
                n254 = property on="3 3" class="Bool (严格)"("Colors [4]"=w52) -> ()  [unwired: 2 in, 2 out]
                n255 = property on="4 3" class="Bool (严格)"("Colors [4]"=w51) -> ()  [unwired: 2 in, 2 out]
                n256 = property on="5 3" class="Bool (严格)"("Colors [4]"=w51) -> ()  [unwired: 2 in, 2 out]
                n257 = property on="1 3" class="Bool (严格)"("Colors [4]"=w51) -> ()  [unwired: 2 in, 2 out]
                n258 = property on="2 3" class="Bool (严格)"("Colors [4]"=w51) -> ()  [unwired: 2 in, 2 out]
              }
              frame 3 {
                n259 = property on="6 3" class="Bool (严格)"("Colors [4]"=w54) -> ()  [unwired: 2 in, 2 out]
                n260 = property on="7 3" class="Bool (严格)"("Colors [4]"=w53) -> ()  [unwired: 2 in, 2 out]
                n261 = property on="3 3" class="Bool (严格)"("Colors [4]"=w53) -> ()  [unwired: 2 in, 2 out]
                n262 = property on="4 3" class="Bool (严格)"("Colors [4]"=w53) -> ()  [unwired: 2 in, 2 out]
                n263 = property on="5 3" class="Bool (严格)"("Colors [4]"=w54) -> ()  [unwired: 2 in, 2 out]
                n264 = property on="1 3" class="Bool (严格)"("Colors [4]"=w53) -> ()  [unwired: 2 in, 2 out]
                n265 = property on="2 3" class="Bool (严格)"("Colors [4]"=w53) -> ()  [unwired: 2 in, 2 out]
              }
              frame 4 {
                n266 = property on="6 3" class="Bool (严格)"("Colors [4]"=w55) -> ()  [unwired: 2 in, 2 out]
                n267 = property on="7 3" class="Bool (严格)"("Colors [4]"=w55) -> ()  [unwired: 2 in, 2 out]
                n268 = property on="3 3" class="Bool (严格)"("Colors [4]"=w55) -> ()  [unwired: 2 in, 2 out]
                n269 = property on="4 3" class="Bool (严格)"("Colors [4]"=w56) -> ()  [unwired: 2 in, 2 out]
                n270 = property on="5 3" class="Bool (严格)"("Colors [4]"=w56) -> ()  [unwired: 2 in, 2 out]
                n271 = property on="1 3" class="Bool (严格)"("Colors [4]"=w56) -> ()  [unwired: 2 in, 2 out]
                n272 = property on="2 3" class="Bool (严格)"("Colors [4]"=w55) -> ()  [unwired: 2 in, 2 out]
              }
              frame 5 {
                n273 = property on="6 3" class="Bool (严格)"("Colors [4]"=w57) -> ()  [unwired: 2 in, 2 out]
                n274 = property on="7 3" class="Bool (严格)"("Colors [4]"=w57) -> ()  [unwired: 2 in, 2 out]
                n275 = property on="3 3" class="Bool (严格)"("Colors [4]"=w57) -> ()  [unwired: 2 in, 2 out]
                n276 = property on="4 3" class="Bool (严格)"("Colors [4]"=w57) -> ()  [unwired: 2 in, 2 out]
                n277 = property on="5 3" class="Bool (严格)"("Colors [4]"=w58) -> ()  [unwired: 2 in, 2 out]
                n278 = property on="1 3" class="Bool (严格)"("Colors [4]"=w57) -> ()  [unwired: 2 in, 2 out]
                n279 = property on="2 3" class="Bool (严格)"("Colors [4]"=w58) -> ()  [unwired: 2 in, 2 out]
              }
              frame 6 {
                n280 = property on="6 3" class="Bool (严格)"("Colors [4]"=w59) -> ()  [unwired: 2 in, 2 out]
                n281 = property on="7 3" class="Bool (严格)"("Colors [4]"=w59) -> ()  [unwired: 2 in, 2 out]
                n282 = property on="3 3" class="Bool (严格)"("Colors [4]"=w59) -> ()  [unwired: 2 in, 2 out]
                n283 = property on="4 3" class="Bool (严格)"("Colors [4]"=w59) -> ()  [unwired: 2 in, 2 out]
                n284 = property on="5 3" class="Bool (严格)"("Colors [4]"=w59) -> ()  [unwired: 2 in, 2 out]
                n285 = property on="1 3" class="Bool (严格)"("Colors [4]"=w59) -> ()  [unwired: 2 in, 2 out]
                n286 = property on="2 3" class="Bool (严格)"("Colors [4]"=w60) -> ()  [unwired: 2 in, 2 out]
              }
              frame 7 {
                n287 = property on="6 3" class="Bool (严格)"("Colors [4]"=w61) -> ()  [unwired: 2 in, 2 out]
                n288 = property on="7 3" class="Bool (严格)"("Colors [4]"=w61) -> ()  [unwired: 2 in, 2 out]
                n289 = property on="3 3" class="Bool (严格)"("Colors [4]"=w62) -> ()  [unwired: 2 in, 2 out]
                n290 = property on="4 3" class="Bool (严格)"("Colors [4]"=w61) -> ()  [unwired: 2 in, 2 out]
                n291 = property on="5 3" class="Bool (严格)"("Colors [4]"=w61) -> ()  [unwired: 2 in, 2 out]
                n292 = property on="1 3" class="Bool (严格)"("Colors [4]"=w62) -> ()  [unwired: 2 in, 2 out]
                n293 = property on="2 3" class="Bool (严格)"("Colors [4]"=w62) -> ()  [unwired: 2 in, 2 out]
              }
              frame 8 {
                n294 = property on="6 3" class="Bool (严格)"("Colors [4]"=w63) -> ()  [unwired: 2 in, 2 out]
                n295 = property on="7 3" class="Bool (严格)"("Colors [4]"=w63) -> ()  [unwired: 2 in, 2 out]
                n296 = property on="3 3" class="Bool (严格)"("Colors [4]"=w63) -> ()  [unwired: 2 in, 2 out]
                n297 = property on="4 3" class="Bool (严格)"("Colors [4]"=w63) -> ()  [unwired: 2 in, 2 out]
                n298 = property on="5 3" class="Bool (严格)"("Colors [4]"=w63) -> ()  [unwired: 2 in, 2 out]
                n299 = property on="1 3" class="Bool (严格)"("Colors [4]"=w63) -> ()  [unwired: 2 in, 2 out]
                n300 = property on="2 3" class="Bool (严格)"("Colors [4]"=w63) -> ()  [unwired: 2 in, 2 out]
              }
              frame 9 {
                n301 = property on="6 3" class="Bool (严格)"("Colors [4]"=w64) -> ()  [unwired: 2 in, 2 out]
                n302 = property on="7 3" class="Bool (严格)"("Colors [4]"=w64) -> ()  [unwired: 2 in, 2 out]
                n303 = property on="3 3" class="Bool (严格)"("Colors [4]"=w64) -> ()  [unwired: 2 in, 2 out]
                n304 = property on="4 3" class="Bool (严格)"("Colors [4]"=w64) -> ()  [unwired: 2 in, 2 out]
                n305 = property on="5 3" class="Bool (严格)"("Colors [4]"=w65) -> ()  [unwired: 2 in, 2 out]
                n306 = property on="1 3" class="Bool (严格)"("Colors [4]"=w64) -> ()  [unwired: 2 in, 2 out]
                n307 = property on="2 3" class="Bool (严格)"("Colors [4]"=w64) -> ()  [unwired: 2 in, 2 out]
              }
            }
            n308 = case shown="1" w46 {
              tunnel: cluster{u32, u32}[] [{16715776, 16715776}] ("颜色[4]") -> [w67 w68 w71 w72]
              tunnel: cluster{u32, u32}[] [{16777216, 16777216}] ("颜色[4]") -> [w66 w69 w70 w73]
              frame 0, Default {
                n309 = property on="1 2" class="Bool (严格)"("Colors [4]"=w67) -> ()  [unwired: 2 in, 2 out]
                n310 = property on="2 2" class="Bool (严格)"("Colors [4]"=w67) -> ()  [unwired: 2 in, 2 out]
                n311 = property on="3 2" class="Bool (严格)"("Colors [4]"=w67) -> ()  [unwired: 2 in, 2 out]
                n312 = property on="4 2" class="Bool (严格)"("Colors [4]"=w67) -> ()  [unwired: 2 in, 2 out]
                n313 = property on="5 2" class="Bool (严格)"("Colors [4]"=w67) -> ()  [unwired: 2 in, 2 out]
                n314 = property on="6 2" class="Bool (严格)"("Colors [4]"=w67) -> ()  [unwired: 2 in, 2 out]
                n315 = property on="7 2" class="Bool (严格)"("Colors [4]"=w66) -> ()  [unwired: 2 in, 2 out]
              }
              frame 1 {
                n316 = property on="1 2" class="Bool (严格)"("Colors [4]"=w69) -> ()  [unwired: 2 in, 2 out]
                n317 = property on="2 2" class="Bool (严格)"("Colors [4]"=w68) -> ()  [unwired: 2 in, 2 out]
                n318 = property on="3 2" class="Bool (严格)"("Colors [4]"=w68) -> ()  [unwired: 2 in, 2 out]
                n319 = property on="4 2" class="Bool (严格)"("Colors [4]"=w69) -> ()  [unwired: 2 in, 2 out]
                n320 = property on="5 2" class="Bool (严格)"("Colors [4]"=w69) -> ()  [unwired: 2 in, 2 out]
                n321 = property on="6 2" class="Bool (严格)"("Colors [4]"=w69) -> ()  [unwired: 2 in, 2 out]
                n322 = property on="7 2" class="Bool (严格)"("Colors [4]"=w69) -> ()  [unwired: 2 in, 2 out]
              }
              frame 2 {
                n323 = property on="1 2" class="Bool (严格)"("Colors [4]"=w71) -> ()  [unwired: 2 in, 2 out]
                n324 = property on="2 2" class="Bool (严格)"("Colors [4]"=w71) -> ()  [unwired: 2 in, 2 out]
                n325 = property on="3 2" class="Bool (严格)"("Colors [4]"=w70) -> ()  [unwired: 2 in, 2 out]
                n326 = property on="4 2" class="Bool (严格)"("Colors [4]"=w71) -> ()  [unwired: 2 in, 2 out]
                n327 = property on="5 2" class="Bool (严格)"("Colors [4]"=w71) -> ()  [unwired: 2 in, 2 out]
                n328 = property on="6 2" class="Bool (严格)"("Colors [4]"=w70) -> ()  [unwired: 2 in, 2 out]
                n329 = property on="7 2" class="Bool (严格)"("Colors [4]"=w71) -> ()  [unwired: 2 in, 2 out]
              }
              frame 3 {
                n330 = property on="1 2" class="Bool (严格)"("Colors [4]"=w72) -> ()  [unwired: 2 in, 2 out]
                n331 = property on="2 2" class="Bool (严格)"("Colors [4]"=w72) -> ()  [unwired: 2 in, 2 out]
                n332 = property on="3 2" class="Bool (严格)"("Colors [4]"=w72) -> ()  [unwired: 2 in, 2 out]
                n333 = property on="4 2" class="Bool (严格)"("Colors [4]"=w72) -> ()  [unwired: 2 in, 2 out]
                n334 = property on="5 2" class="Bool (严格)"("Colors [4]"=w73) -> ()  [unwired: 2 in, 2 out]
                n335 = property on="6 2" class="Bool (严格)"("Colors [4]"=w73) -> ()  [unwired: 2 in, 2 out]
                n336 = property on="7 2" class="Bool (严格)"("Colors [4]"=w72) -> ()  [unwired: 2 in, 2 out]
              }
            }
          }
          frame True {
            n337 = Quotient & Remainder(x=w77, y=100.0) -> (x-y*floor(x/y)=w82:dbl)  [unwired: 1 out]
            n338 = Quotient & Remainder(x=w82, y=10.0) -> (x-y*floor(x/y)=w74:dbl, floor(x/y)=w83:dbl)
            n339 = case shown="1" w83 {
              tunnel: cluster{u32, u32}[] [{65379, 65379}] ("颜色[4]") -> [w104 w105 w108 w109 w111 w113 w115 w118 w119 w120]
              tunnel: cluster{u32, u32}[] [{16777216, 16777216}] ("颜色[4]") -> [w103 w106 w107 w110 w112 w114 w116 w117 _ w121]
              frame 0, Default {
                n340 = property on="1 2" class="Bool (严格)"("Colors [4]"=w104) -> ()  [unwired: 2 in, 2 out]
                n341 = property on="2 2" class="Bool (严格)"("Colors [4]"=w104) -> ()  [unwired: 2 in, 2 out]
                n342 = property on="3 2" class="Bool (严格)"("Colors [4]"=w104) -> ()  [unwired: 2 in, 2 out]
                n343 = property on="4 2" class="Bool (严格)"("Colors [4]"=w104) -> ()  [unwired: 2 in, 2 out]
                n344 = property on="5 2" class="Bool (严格)"("Colors [4]"=w104) -> ()  [unwired: 2 in, 2 out]
                n345 = property on="6 2" class="Bool (严格)"("Colors [4]"=w104) -> ()  [unwired: 2 in, 2 out]
                n346 = property on="7 2" class="Bool (严格)"("Colors [4]"=w103) -> ()  [unwired: 2 in, 2 out]
              }
              frame 1 {
                n347 = property on="1 2" class="Bool (严格)"("Colors [4]"=w106) -> ()  [unwired: 2 in, 2 out]
                n348 = property on="2 2" class="Bool (严格)"("Colors [4]"=w105) -> ()  [unwired: 2 in, 2 out]
                n349 = property on="3 2" class="Bool (严格)"("Colors [4]"=w105) -> ()  [unwired: 2 in, 2 out]
                n350 = property on="4 2" class="Bool (严格)"("Colors [4]"=w106) -> ()  [unwired: 2 in, 2 out]
                n351 = property on="5 2" class="Bool (严格)"("Colors [4]"=w106) -> ()  [unwired: 2 in, 2 out]
                n352 = property on="6 2" class="Bool (严格)"("Colors [4]"=w106) -> ()  [unwired: 2 in, 2 out]
                n353 = property on="7 2" class="Bool (严格)"("Colors [4]"=w106) -> ()  [unwired: 2 in, 2 out]
              }
              frame 2 {
                n354 = property on="1 2" class="Bool (严格)"("Colors [4]"=w108) -> ()  [unwired: 2 in, 2 out]
                n355 = property on="2 2" class="Bool (严格)"("Colors [4]"=w108) -> ()  [unwired: 2 in, 2 out]
                n356 = property on="3 2" class="Bool (严格)"("Colors [4]"=w107) -> ()  [unwired: 2 in, 2 out]
                n357 = property on="4 2" class="Bool (严格)"("Colors [4]"=w108) -> ()  [unwired: 2 in, 2 out]
                n358 = property on="5 2" class="Bool (严格)"("Colors [4]"=w108) -> ()  [unwired: 2 in, 2 out]
                n359 = property on="6 2" class="Bool (严格)"("Colors [4]"=w107) -> ()  [unwired: 2 in, 2 out]
                n360 = property on="7 2" class="Bool (严格)"("Colors [4]"=w108) -> ()  [unwired: 2 in, 2 out]
              }
              frame 3 {
                n361 = property on="1 2" class="Bool (严格)"("Colors [4]"=w109) -> ()  [unwired: 2 in, 2 out]
                n362 = property on="2 2" class="Bool (严格)"("Colors [4]"=w109) -> ()  [unwired: 2 in, 2 out]
                n363 = property on="3 2" class="Bool (严格)"("Colors [4]"=w109) -> ()  [unwired: 2 in, 2 out]
                n364 = property on="4 2" class="Bool (严格)"("Colors [4]"=w109) -> ()  [unwired: 2 in, 2 out]
                n365 = property on="5 2" class="Bool (严格)"("Colors [4]"=w110) -> ()  [unwired: 2 in, 2 out]
                n366 = property on="6 2" class="Bool (严格)"("Colors [4]"=w110) -> ()  [unwired: 2 in, 2 out]
                n367 = property on="7 2" class="Bool (严格)"("Colors [4]"=w109) -> ()  [unwired: 2 in, 2 out]
              }
              frame 4 {
                n368 = property on="1 2" class="Bool (严格)"("Colors [4]"=w112) -> ()  [unwired: 2 in, 2 out]
                n369 = property on="2 2" class="Bool (严格)"("Colors [4]"=w111) -> ()  [unwired: 2 in, 2 out]
                n370 = property on="3 2" class="Bool (严格)"("Colors [4]"=w111) -> ()  [unwired: 2 in, 2 out]
                n371 = property on="4 2" class="Bool (严格)"("Colors [4]"=w112) -> ()  [unwired: 2 in, 2 out]
                n372 = property on="5 2" class="Bool (严格)"("Colors [4]"=w112) -> ()  [unwired: 2 in, 2 out]
                n373 = property on="6 2" class="Bool (严格)"("Colors [4]"=w111) -> ()  [unwired: 2 in, 2 out]
                n374 = property on="7 2" class="Bool (严格)"("Colors [4]"=w111) -> ()  [unwired: 2 in, 2 out]
              }
              frame 5 {
                n375 = property on="1 2" class="Bool (严格)"("Colors [4]"=w113) -> ()  [unwired: 2 in, 2 out]
                n376 = property on="2 2" class="Bool (严格)"("Colors [4]"=w114) -> ()  [unwired: 2 in, 2 out]
                n377 = property on="3 2" class="Bool (严格)"("Colors [4]"=w113) -> ()  [unwired: 2 in, 2 out]
                n378 = property on="4 2" class="Bool (严格)"("Colors [4]"=w113) -> ()  [unwired: 2 in, 2 out]
                n379 = property on="5 2" class="Bool (严格)"("Colors [4]"=w114) -> ()  [unwired: 2 in, 2 out]
                n380 = property on="6 2" class="Bool (严格)"("Colors [4]"=w113) -> ()  [unwired: 2 in, 2 out]
                n381 = property on="7 2" class="Bool (严格)"("Colors [4]"=w113) -> ()  [unwired: 2 in, 2 out]
              }
              frame 6 {
                n382 = property on="1 2" class="Bool (严格)"("Colors [4]"=w115) -> ()  [unwired: 2 in, 2 out]
                n383 = property on="2 2" class="Bool (严格)"("Colors [4]"=w116) -> ()  [unwired: 2 in, 2 out]
                n384 = property on="3 2" class="Bool (严格)"("Colors [4]"=w115) -> ()  [unwired: 2 in, 2 out]
                n385 = property on="4 2" class="Bool (严格)"("Colors [4]"=w115) -> ()  [unwired: 2 in, 2 out]
                n386 = property on="5 2" class="Bool (严格)"("Colors [4]"=w115) -> ()  [unwired: 2 in, 2 out]
                n387 = property on="6 2" class="Bool (严格)"("Colors [4]"=w115) -> ()  [unwired: 2 in, 2 out]
                n388 = property on="7 2" class="Bool (严格)"("Colors [4]"=w115) -> ()  [unwired: 2 in, 2 out]
              }
              frame 7 {
                n389 = property on="1 2" class="Bool (严格)"("Colors [4]"=w118) -> ()  [unwired: 2 in, 2 out]
                n390 = property on="2 2" class="Bool (严格)"("Colors [4]"=w118) -> ()  [unwired: 2 in, 2 out]
                n391 = property on="3 2" class="Bool (严格)"("Colors [4]"=w118) -> ()  [unwired: 2 in, 2 out]
                n392 = property on="4 2" class="Bool (严格)"("Colors [4]"=w117) -> ()  [unwired: 2 in, 2 out]
                n393 = property on="5 2" class="Bool (严格)"("Colors [4]"=w117) -> ()  [unwired: 2 in, 2 out]
                n394 = property on="6 2" class="Bool (严格)"("Colors [4]"=w117) -> ()  [unwired: 2 in, 2 out]
                n395 = property on="7 2" class="Bool (严格)"("Colors [4]"=w117) -> ()  [unwired: 2 in, 2 out]
              }
              frame 8 {
                n396 = property on="1 2" class="Bool (严格)"("Colors [4]"=w119) -> ()  [unwired: 2 in, 2 out]
                n397 = property on="2 2" class="Bool (严格)"("Colors [4]"=w119) -> ()  [unwired: 2 in, 2 out]
                n398 = property on="3 2" class="Bool (严格)"("Colors [4]"=w119) -> ()  [unwired: 2 in, 2 out]
                n399 = property on="4 2" class="Bool (严格)"("Colors [4]"=w119) -> ()  [unwired: 2 in, 2 out]
                n400 = property on="5 2" class="Bool (严格)"("Colors [4]"=w119) -> ()  [unwired: 2 in, 2 out]
                n401 = property on="6 2" class="Bool (严格)"("Colors [4]"=w119) -> ()  [unwired: 2 in, 2 out]
                n402 = property on="7 2" class="Bool (严格)"("Colors [4]"=w119) -> ()  [unwired: 2 in, 2 out]
              }
              frame 9 {
                n403 = property on="1 2" class="Bool (严格)"("Colors [4]"=w120) -> ()  [unwired: 2 in, 2 out]
                n404 = property on="2 2" class="Bool (严格)"("Colors [4]"=w120) -> ()  [unwired: 2 in, 2 out]
                n405 = property on="3 2" class="Bool (严格)"("Colors [4]"=w120) -> ()  [unwired: 2 in, 2 out]
                n406 = property on="4 2" class="Bool (严格)"("Colors [4]"=w120) -> ()  [unwired: 2 in, 2 out]
                n407 = property on="5 2" class="Bool (严格)"("Colors [4]"=w121) -> ()  [unwired: 2 in, 2 out]
                n408 = property on="6 2" class="Bool (严格)"("Colors [4]"=w120) -> ()  [unwired: 2 in, 2 out]
                n409 = property on="7 2" class="Bool (严格)"("Colors [4]"=w120) -> ()  [unwired: 2 in, 2 out]
              }
            }
            n410 = case shown="6" w74 {
              tunnel: cluster{u32, u32}[] [{65379, 65379}] ("颜色[4]") -> [w85 w87 w88 w90 w92 w94 w96 w99 w100 w101]
              tunnel: cluster{u32, u32}[] [{16777216, 16777216}] ("颜色[4]") -> [w84 w86 w89 w91 w93 w95 w97 w98 _ w102]
              frame 0, Default {
                n411 = property on="6 3" class="Bool (严格)"("Colors [4]"=w85) -> ()  [unwired: 2 in, 2 out]
                n412 = property on="7 3" class="Bool (严格)"("Colors [4]"=w84) -> ()  [unwired: 2 in, 2 out]
                n413 = property on="3 3" class="Bool (严格)"("Colors [4]"=w85) -> ()  [unwired: 2 in, 2 out]
                n414 = property on="4 3" class="Bool (严格)"("Colors [4]"=w85) -> ()  [unwired: 2 in, 2 out]
                n415 = property on="5 3" class="Bool (严格)"("Colors [4]"=w85) -> ()  [unwired: 2 in, 2 out]
                n416 = property on="1 3" class="Bool (严格)"("Colors [4]"=w85) -> ()  [unwired: 2 in, 2 out]
                n417 = property on="2 3" class="Bool (严格)"("Colors [4]"=w85) -> ()  [unwired: 2 in, 2 out]
              }
              frame 1 {
                n418 = property on="6 3" class="Bool (严格)"("Colors [4]"=w86) -> ()  [unwired: 2 in, 2 out]
                n419 = property on="7 3" class="Bool (严格)"("Colors [4]"=w86) -> ()  [unwired: 2 in, 2 out]
                n420 = property on="3 3" class="Bool (严格)"("Colors [4]"=w87) -> ()  [unwired: 2 in, 2 out]
                n421 = property on="4 3" class="Bool (严格)"("Colors [4]"=w86) -> ()  [unwired: 2 in, 2 out]
                n422 = property on="5 3" class="Bool (严格)"("Colors [4]"=w86) -> ()  [unwired: 2 in, 2 out]
                n423 = property on="1 3" class="Bool (严格)"("Colors [4]"=w86) -> ()  [unwired: 2 in, 2 out]
                n424 = property on="2 3" class="Bool (严格)"("Colors [4]"=w87) -> ()  [unwired: 2 in, 2 out]
              }
              frame 2 {
                n425 = property on="6 3" class="Bool (严格)"("Colors [4]"=w89) -> ()  [unwired: 2 in, 2 out]
                n426 = property on="7 3" class="Bool (严格)"("Colors [4]"=w88) -> ()  [unwired: 2 in, 2 out]
                n427 = property on="3 3" class="Bool (严格)"("Colors [4]"=w89) -> ()  [unwired: 2 in, 2 out]
                n428 = property on="4 3" class="Bool (严格)"("Colors [4]"=w88) -> ()  [unwired: 2 in, 2 out]
                n429 = property on="5 3" class="Bool (严格)"("Colors [4]"=w88) -> ()  [unwired: 2 in, 2 out]
                n430 = property on="1 3" class="Bool (严格)"("Colors [4]"=w88) -> ()  [unwired: 2 in, 2 out]
                n431 = property on="2 3" class="Bool (严格)"("Colors [4]"=w88) -> ()  [unwired: 2 in, 2 out]
              }
              frame 3 {
                n432 = property on="6 3" class="Bool (严格)"("Colors [4]"=w91) -> ()  [unwired: 2 in, 2 out]
                n433 = property on="7 3" class="Bool (严格)"("Colors [4]"=w90) -> ()  [unwired: 2 in, 2 out]
                n434 = property on="3 3" class="Bool (严格)"("Colors [4]"=w90) -> ()  [unwired: 2 in, 2 out]
                n435 = property on="4 3" class="Bool (严格)"("Colors [4]"=w90) -> ()  [unwired: 2 in, 2 out]
                n436 = property on="5 3" class="Bool (严格)"("Colors [4]"=w91) -> ()  [unwired: 2 in, 2 out]
                n437 = property on="1 3" class="Bool (严格)"("Colors [4]"=w90) -> ()  [unwired: 2 in, 2 out]
                n438 = property on="2 3" class="Bool (严格)"("Colors [4]"=w90) -> ()  [unwired: 2 in, 2 out]
              }
              frame 4 {
                n439 = property on="6 3" class="Bool (严格)"("Colors [4]"=w92) -> ()  [unwired: 2 in, 2 out]
                n440 = property on="7 3" class="Bool (严格)"("Colors [4]"=w92) -> ()  [unwired: 2 in, 2 out]
                n441 = property on="3 3" class="Bool (严格)"("Colors [4]"=w92) -> ()  [unwired: 2 in, 2 out]
                n442 = property on="4 3" class="Bool (严格)"("Colors [4]"=w93) -> ()  [unwired: 2 in, 2 out]
                n443 = property on="5 3" class="Bool (严格)"("Colors [4]"=w93) -> ()  [unwired: 2 in, 2 out]
                n444 = property on="1 3" class="Bool (严格)"("Colors [4]"=w93) -> ()  [unwired: 2 in, 2 out]
                n445 = property on="2 3" class="Bool (严格)"("Colors [4]"=w92) -> ()  [unwired: 2 in, 2 out]
              }
              frame 5 {
                n446 = property on="6 3" class="Bool (严格)"("Colors [4]"=w94) -> ()  [unwired: 2 in, 2 out]
                n447 = property on="7 3" class="Bool (严格)"("Colors [4]"=w94) -> ()  [unwired: 2 in, 2 out]
                n448 = property on="3 3" class="Bool (严格)"("Colors [4]"=w94) -> ()  [unwired: 2 in, 2 out]
                n449 = property on="4 3" class="Bool (严格)"("Colors [4]"=w94) -> ()  [unwired: 2 in, 2 out]
                n450 = property on="5 3" class="Bool (严格)"("Colors [4]"=w95) -> ()  [unwired: 2 in, 2 out]
                n451 = property on="1 3" class="Bool (严格)"("Colors [4]"=w94) -> ()  [unwired: 2 in, 2 out]
                n452 = property on="2 3" class="Bool (严格)"("Colors [4]"=w95) -> ()  [unwired: 2 in, 2 out]
              }
              frame 6 {
                n453 = property on="6 3" class="Bool (严格)"("Colors [4]"=w96) -> ()  [unwired: 2 in, 2 out]
                n454 = property on="7 3" class="Bool (严格)"("Colors [4]"=w96) -> ()  [unwired: 2 in, 2 out]
                n455 = property on="3 3" class="Bool (严格)"("Colors [4]"=w96) -> ()  [unwired: 2 in, 2 out]
                n456 = property on="4 3" class="Bool (严格)"("Colors [4]"=w96) -> ()  [unwired: 2 in, 2 out]
                n457 = property on="5 3" class="Bool (严格)"("Colors [4]"=w96) -> ()  [unwired: 2 in, 2 out]
                n458 = property on="1 3" class="Bool (严格)"("Colors [4]"=w96) -> ()  [unwired: 2 in, 2 out]
                n459 = property on="2 3" class="Bool (严格)"("Colors [4]"=w97) -> ()  [unwired: 2 in, 2 out]
              }
              frame 7 {
                n460 = property on="6 3" class="Bool (严格)"("Colors [4]"=w98) -> ()  [unwired: 2 in, 2 out]
                n461 = property on="7 3" class="Bool (严格)"("Colors [4]"=w98) -> ()  [unwired: 2 in, 2 out]
                n462 = property on="3 3" class="Bool (严格)"("Colors [4]"=w99) -> ()  [unwired: 2 in, 2 out]
                n463 = property on="4 3" class="Bool (严格)"("Colors [4]"=w98) -> ()  [unwired: 2 in, 2 out]
                n464 = property on="5 3" class="Bool (严格)"("Colors [4]"=w98) -> ()  [unwired: 2 in, 2 out]
                n465 = property on="1 3" class="Bool (严格)"("Colors [4]"=w99) -> ()  [unwired: 2 in, 2 out]
                n466 = property on="2 3" class="Bool (严格)"("Colors [4]"=w99) -> ()  [unwired: 2 in, 2 out]
              }
              frame 8 {
                n467 = property on="6 3" class="Bool (严格)"("Colors [4]"=w100) -> ()  [unwired: 2 in, 2 out]
                n468 = property on="7 3" class="Bool (严格)"("Colors [4]"=w100) -> ()  [unwired: 2 in, 2 out]
                n469 = property on="3 3" class="Bool (严格)"("Colors [4]"=w100) -> ()  [unwired: 2 in, 2 out]
                n470 = property on="4 3" class="Bool (严格)"("Colors [4]"=w100) -> ()  [unwired: 2 in, 2 out]
                n471 = property on="5 3" class="Bool (严格)"("Colors [4]"=w100) -> ()  [unwired: 2 in, 2 out]
                n472 = property on="1 3" class="Bool (严格)"("Colors [4]"=w100) -> ()  [unwired: 2 in, 2 out]
                n473 = property on="2 3" class="Bool (严格)"("Colors [4]"=w100) -> ()  [unwired: 2 in, 2 out]
              }
              frame 9 {
                n474 = property on="6 3" class="Bool (严格)"("Colors [4]"=w101) -> ()  [unwired: 2 in, 2 out]
                n475 = property on="7 3" class="Bool (严格)"("Colors [4]"=w101) -> ()  [unwired: 2 in, 2 out]
                n476 = property on="3 3" class="Bool (严格)"("Colors [4]"=w101) -> ()  [unwired: 2 in, 2 out]
                n477 = property on="4 3" class="Bool (严格)"("Colors [4]"=w101) -> ()  [unwired: 2 in, 2 out]
                n478 = property on="5 3" class="Bool (严格)"("Colors [4]"=w102) -> ()  [unwired: 2 in, 2 out]
                n479 = property on="1 3" class="Bool (严格)"("Colors [4]"=w101) -> ()  [unwired: 2 in, 2 out]
                n480 = property on="2 3" class="Bool (严格)"("Colors [4]"=w101) -> ()  [unwired: 2 in, 2 out]
              }
            }
          }
        }
      }
      frame 10 {
        n481 = Quotient & Remainder(x=w190, y=10) -> (x-y*floor(x/y)=w191:i32, floor(x/y)=w194:i32)
        n482 = case shown="0, 默认" w191 {
          tunnel: [T2 {"7"=TRUE, "6"=TRUE, "5"=TRUE, "4"=TRUE, "3"=TRUE, "2"=TRUE, "1"=FALSE} ("簇") T2 {"7"=FALSE, "6"=TRUE, "5"=TRUE, "4"=FALSE, "3"=FALSE, "2"=FALSE, "1"=FALSE} ("簇") T2 {"7"=TRUE, "6"=TRUE, "5"=FALSE, "4"=TRUE, "3"=TRUE, "2"=FALSE, "1"=TRUE} ("簇") T2 {"7"=TRUE, "6"=TRUE, "5"=TRUE, "4"=TRUE, "3"=FALSE, "2"=FALSE, "1"=TRUE} ("簇") T2 {"7"=FALSE, "6"=TRUE, "5"=TRUE, "4"=FALSE, "3"=FALSE, "2"=TRUE, "1"=TRUE} ("簇") T2 {"7"=TRUE, "6"=FALSE, "5"=TRUE, "4"=TRUE, "3"=FALSE, "2"=TRUE, "1"=TRUE} ("簇") T2 {"7"=TRUE, "6"=FALSE, "5"=TRUE, "4"=TRUE, "3"=TRUE, "2"=TRUE, "1"=TRUE} ("簇") T2 {"7"=TRUE, "6"=TRUE, "5"=TRUE, "4"=FALSE, "3"=FALSE, "2"=FALSE, "1"=FALSE} ("簇") T2 {"7"=TRUE, "6"=TRUE, "5"=TRUE, "4"=TRUE, "3"=TRUE, "2"=TRUE, "1"=TRUE} ("簇") T2 {"7"=TRUE, "6"=TRUE, "5"=TRUE, "4"=TRUE, "3"=FALSE, "2"=TRUE, "1"=TRUE} ("簇")] -> w192
          frame 0, Default {
          }
          frame 1 {
          }
          frame 2 {
          }
          frame 3 {
          }
          frame 4 {
          }
          frame 5 {
          }
          frame 6 {
          }
          frame 7 {
          }
          frame 8 {
          }
          frame 9 {
          }
        }
        "红方本局得分个位" <- w192
        n483 = case shown="0, 默认" w194 {
          tunnel: [T2 {"7"=TRUE, "6"=TRUE, "5"=TRUE, "4"=TRUE, "3"=TRUE, "2"=TRUE, "1"=FALSE} ("簇") T2 {"7"=FALSE, "6"=TRUE, "5"=TRUE, "4"=FALSE, "3"=FALSE, "2"=FALSE, "1"=FALSE} ("簇") T2 {"7"=TRUE, "6"=TRUE, "5"=FALSE, "4"=TRUE, "3"=TRUE, "2"=FALSE, "1"=TRUE} ("簇") T2 {"7"=TRUE, "6"=TRUE, "5"=TRUE, "4"=TRUE, "3"=FALSE, "2"=FALSE, "1"=TRUE} ("簇") T2 {"7"=FALSE, "6"=TRUE, "5"=TRUE, "4"=FALSE, "3"=FALSE, "2"=TRUE, "1"=TRUE} ("簇") T2 {"7"=TRUE, "6"=FALSE, "5"=TRUE, "4"=TRUE, "3"=FALSE, "2"=TRUE, "1"=TRUE} ("簇") T2 {"7"=TRUE, "6"=FALSE, "5"=TRUE, "4"=TRUE, "3"=TRUE, "2"=TRUE, "1"=TRUE} ("簇") T2 {"7"=TRUE, "6"=TRUE, "5"=TRUE, "4"=FALSE, "3"=FALSE, "2"=FALSE, "1"=FALSE} ("簇") T2 {"7"=TRUE, "6"=TRUE, "5"=TRUE, "4"=TRUE, "3"=TRUE, "2"=TRUE, "1"=TRUE} ("簇") T2 {"7"=TRUE, "6"=TRUE, "5"=TRUE, "4"=TRUE, "3"=FALSE, "2"=TRUE, "1"=TRUE} ("簇")] -> w193
          frame 0, Default {
          }
          frame 1 {
          }
          frame 2 {
          }
          frame 3 {
          }
          frame 4 {
          }
          frame 5 {
          }
          frame 6 {
          }
          frame 7 {
          }
          frame 8 {
          }
          frame 9 {
          }
        }
        "红方本局得分十位" <- w193
      }
      frame 11 {
        n484 = Quotient & Remainder(x=w219, y=10) -> (x-y*floor(x/y)=w217:i32, floor(x/y)=w218:i32)
        n485 = case shown="3" w217 {
          tunnel: [T2 {"7"=TRUE, "6"=TRUE, "5"=TRUE, "4"=TRUE, "3"=TRUE, "2"=TRUE, "1"=FALSE} ("簇") T2 {"7"=FALSE, "6"=TRUE, "5"=TRUE, "4"=FALSE, "3"=FALSE, "2"=FALSE, "1"=FALSE} ("簇") T2 {"7"=TRUE, "6"=TRUE, "5"=FALSE, "4"=TRUE, "3"=TRUE, "2"=FALSE, "1"=TRUE} ("簇") T2 {"7"=TRUE, "6"=TRUE, "5"=TRUE, "4"=TRUE, "3"=FALSE, "2"=FALSE, "1"=TRUE} ("簇") T2 {"7"=FALSE, "6"=TRUE, "5"=TRUE, "4"=FALSE, "3"=FALSE, "2"=TRUE, "1"=TRUE} ("簇") T2 {"7"=TRUE, "6"=FALSE, "5"=TRUE, "4"=TRUE, "3"=FALSE, "2"=TRUE, "1"=TRUE} ("簇") T2 {"7"=TRUE, "6"=FALSE, "5"=TRUE, "4"=TRUE, "3"=TRUE, "2"=TRUE, "1"=TRUE} ("簇") T2 {"7"=TRUE, "6"=TRUE, "5"=TRUE, "4"=FALSE, "3"=FALSE, "2"=FALSE, "1"=FALSE} ("簇") T2 {"7"=TRUE, "6"=TRUE, "5"=TRUE, "4"=TRUE, "3"=TRUE, "2"=TRUE, "1"=TRUE} ("簇") T2 {"7"=TRUE, "6"=TRUE, "5"=TRUE, "4"=TRUE, "3"=FALSE, "2"=TRUE, "1"=TRUE} ("簇")] -> w216
          frame 0, Default {
          }
          frame 1 {
          }
          frame 2 {
          }
          frame 3 {
          }
          frame 4 {
          }
          frame 5 {
          }
          frame 6 {
          }
          frame 7 {
          }
          frame 8 {
          }
          frame 9 {
          }
        }
        "蓝方本局得分个位" <- w216
        n486 = case shown="3" w218 {
          tunnel: [T2 {"7"=TRUE, "6"=TRUE, "5"=TRUE, "4"=TRUE, "3"=TRUE, "2"=TRUE, "1"=FALSE} ("簇") T2 {"7"=FALSE, "6"=TRUE, "5"=TRUE, "4"=FALSE, "3"=FALSE, "2"=FALSE, "1"=FALSE} ("簇") T2 {"7"=TRUE, "6"=TRUE, "5"=FALSE, "4"=TRUE, "3"=TRUE, "2"=FALSE, "1"=TRUE} ("簇") T2 {"7"=TRUE, "6"=TRUE, "5"=TRUE, "4"=TRUE, "3"=FALSE, "2"=FALSE, "1"=TRUE} ("簇") T2 {"7"=FALSE, "6"=TRUE, "5"=TRUE, "4"=FALSE, "3"=FALSE, "2"=TRUE, "1"=TRUE} ("簇") T2 {"7"=TRUE, "6"=FALSE, "5"=TRUE, "4"=TRUE, "3"=FALSE, "2"=TRUE, "1"=TRUE} ("簇") T2 {"7"=TRUE, "6"=FALSE, "5"=TRUE, "4"=TRUE, "3"=TRUE, "2"=TRUE, "1"=TRUE} ("簇") T2 {"7"=TRUE, "6"=TRUE, "5"=TRUE, "4"=FALSE, "3"=FALSE, "2"=FALSE, "1"=FALSE} ("簇") T2 {"7"=TRUE, "6"=TRUE, "5"=TRUE, "4"=TRUE, "3"=TRUE, "2"=TRUE, "1"=TRUE} ("簇") T2 {"7"=TRUE, "6"=TRUE, "5"=TRUE, "4"=TRUE, "3"=FALSE, "2"=TRUE, "1"=TRUE} ("簇")] -> w221
          frame 0, Default {
          }
          frame 1 {
          }
          frame 2 {
          }
          frame 3 {
          }
          frame 4 {
          }
          frame 5 {
          }
          frame 6 {
          }
          frame 7 {
          }
          frame 8 {
          }
          frame 9 {
          }
        }
        "蓝方本局得分十位" <- w221
      }
      frame 12 {
        n487 = Quotient & Remainder(x=w246, y=10) -> (x-y*floor(x/y)=w242:i32, floor(x/y)=w244:i32)
        n488 = case shown="1" w242 {
          tunnel: [T2 {"7"=TRUE, "6"=TRUE, "5"=TRUE, "4"=TRUE, "3"=TRUE, "2"=TRUE, "1"=FALSE} ("簇") T2 {"7"=FALSE, "6"=TRUE, "5"=TRUE, "4"=FALSE, "3"=FALSE, "2"=FALSE, "1"=FALSE} ("簇") T2 {"7"=TRUE, "6"=TRUE, "5"=FALSE, "4"=TRUE, "3"=TRUE, "2"=FALSE, "1"=TRUE} ("簇") T2 {"7"=TRUE, "6"=TRUE, "5"=TRUE, "4"=TRUE, "3"=FALSE, "2"=FALSE, "1"=TRUE} ("簇") T2 {"7"=FALSE, "6"=TRUE, "5"=TRUE, "4"=FALSE, "3"=FALSE, "2"=TRUE, "1"=TRUE} ("簇") T2 {"7"=TRUE, "6"=FALSE, "5"=TRUE, "4"=TRUE, "3"=FALSE, "2"=TRUE, "1"=TRUE} ("簇") T2 {"7"=TRUE, "6"=FALSE, "5"=TRUE, "4"=TRUE, "3"=TRUE, "2"=TRUE, "1"=TRUE} ("簇") T2 {"7"=TRUE, "6"=TRUE, "5"=TRUE, "4"=FALSE, "3"=FALSE, "2"=FALSE, "1"=FALSE} ("簇") T2 {"7"=TRUE, "6"=TRUE, "5"=TRUE, "4"=TRUE, "3"=TRUE, "2"=TRUE, "1"=TRUE} ("簇") T2 {"7"=TRUE, "6"=TRUE, "5"=TRUE, "4"=TRUE, "3"=FALSE, "2"=TRUE, "1"=TRUE} ("簇")] -> w243
          frame 0, Default {
          }
          frame 1 {
          }
          frame 2 {
          }
          frame 3 {
          }
          frame 4 {
          }
          frame 5 {
          }
          frame 6 {
          }
          frame 7 {
          }
          frame 8 {
          }
          frame 9 {
          }
        }
        "红方胜场比分个位" <- w243
        n489 = case shown="0, 默认" w244 {
          tunnel: [T2 {"7"=TRUE, "6"=TRUE, "5"=TRUE, "4"=TRUE, "3"=TRUE, "2"=TRUE, "1"=FALSE} ("簇") T2 {"7"=FALSE, "6"=TRUE, "5"=TRUE, "4"=FALSE, "3"=FALSE, "2"=FALSE, "1"=FALSE} ("簇") T2 {"7"=TRUE, "6"=TRUE, "5"=FALSE, "4"=TRUE, "3"=TRUE, "2"=FALSE, "1"=TRUE} ("簇") T2 {"7"=TRUE, "6"=TRUE, "5"=TRUE, "4"=TRUE, "3"=FALSE, "2"=FALSE, "1"=TRUE} ("簇") T2 {"7"=FALSE, "6"=TRUE, "5"=TRUE, "4"=FALSE, "3"=FALSE, "2"=TRUE, "1"=TRUE} ("簇") T2 {"7"=TRUE, "6"=FALSE, "5"=TRUE, "4"=TRUE, "3"=FALSE, "2"=TRUE, "1"=TRUE} ("簇") T2 {"7"=TRUE, "6"=FALSE, "5"=TRUE, "4"=TRUE, "3"=TRUE, "2"=TRUE, "1"=TRUE} ("簇") T2 {"7"=TRUE, "6"=TRUE, "5"=TRUE, "4"=FALSE, "3"=FALSE, "2"=FALSE, "1"=FALSE} ("簇") T2 {"7"=TRUE, "6"=TRUE, "5"=TRUE, "4"=TRUE, "3"=TRUE, "2"=TRUE, "1"=TRUE} ("簇") T2 {"7"=TRUE, "6"=TRUE, "5"=TRUE, "4"=TRUE, "3"=FALSE, "2"=TRUE, "1"=TRUE} ("簇")] -> w247
          frame 0, Default {
          }
          frame 1 {
          }
          frame 2 {
          }
          frame 3 {
          }
          frame 4 {
          }
          frame 5 {
          }
          frame 6 {
          }
          frame 7 {
          }
          frame 8 {
          }
          frame 9 {
          }
        }
        "红方胜场比分十位" <- w247
      }
      frame 13 {
        n490 = Quotient & Remainder(x=w271, y=10) -> (x-y*floor(x/y)=w269:i32, floor(x/y)=w268:i32)
        n491 = case shown="3" w269 {
          tunnel: [T2 {"7"=TRUE, "6"=TRUE, "5"=TRUE, "4"=TRUE, "3"=TRUE, "2"=TRUE, "1"=FALSE} ("簇") T2 {"7"=FALSE, "6"=TRUE, "5"=TRUE, "4"=FALSE, "3"=FALSE, "2"=FALSE, "1"=FALSE} ("簇") T2 {"7"=TRUE, "6"=TRUE, "5"=FALSE, "4"=TRUE, "3"=TRUE, "2"=FALSE, "1"=TRUE} ("簇") T2 {"7"=TRUE, "6"=TRUE, "5"=TRUE, "4"=TRUE, "3"=FALSE, "2"=FALSE, "1"=TRUE} ("簇") T2 {"7"=FALSE, "6"=TRUE, "5"=TRUE, "4"=FALSE, "3"=FALSE, "2"=TRUE, "1"=TRUE} ("簇") T2 {"7"=TRUE, "6"=FALSE, "5"=TRUE, "4"=TRUE, "3"=FALSE, "2"=TRUE, "1"=TRUE} ("簇") T2 {"7"=TRUE, "6"=FALSE, "5"=TRUE, "4"=TRUE, "3"=TRUE, "2"=TRUE, "1"=TRUE} ("簇") T2 {"7"=TRUE, "6"=TRUE, "5"=TRUE, "4"=FALSE, "3"=FALSE, "2"=FALSE, "1"=FALSE} ("簇") T2 {"7"=TRUE, "6"=TRUE, "5"=TRUE, "4"=TRUE, "3"=TRUE, "2"=TRUE, "1"=TRUE} ("簇") T2 {"7"=TRUE, "6"=TRUE, "5"=TRUE, "4"=TRUE, "3"=FALSE, "2"=TRUE, "1"=TRUE} ("簇")] -> w272
          frame 0, Default {
          }
          frame 1 {
          }
          frame 2 {
          }
          frame 3 {
          }
          frame 4 {
          }
          frame 5 {
          }
          frame 6 {
          }
          frame 7 {
          }
          frame 8 {
          }
          frame 9 {
          }
        }
        "蓝方胜场得分个位" <- w272
        n492 = case shown="0, 默认" w268 {
          tunnel: [T2 {"7"=TRUE, "6"=TRUE, "5"=TRUE, "4"=TRUE, "3"=TRUE, "2"=TRUE, "1"=FALSE} ("簇") T2 {"7"=FALSE, "6"=TRUE, "5"=TRUE, "4"=FALSE, "3"=FALSE, "2"=FALSE, "1"=FALSE} ("簇") T2 {"7"=TRUE, "6"=TRUE, "5"=FALSE, "4"=TRUE, "3"=TRUE, "2"=FALSE, "1"=TRUE} ("簇") T2 {"7"=TRUE, "6"=TRUE, "5"=TRUE, "4"=TRUE, "3"=FALSE, "2"=FALSE, "1"=TRUE} ("簇") T2 {"7"=FALSE, "6"=TRUE, "5"=TRUE, "4"=FALSE, "3"=FALSE, "2"=TRUE, "1"=TRUE} ("簇") T2 {"7"=TRUE, "6"=FALSE, "5"=TRUE, "4"=TRUE, "3"=FALSE, "2"=TRUE, "1"=TRUE} ("簇") T2 {"7"=TRUE, "6"=FALSE, "5"=TRUE, "4"=TRUE, "3"=TRUE, "2"=TRUE, "1"=TRUE} ("簇") T2 {"7"=TRUE, "6"=TRUE, "5"=TRUE, "4"=FALSE, "3"=FALSE, "2"=FALSE, "1"=FALSE} ("簇") T2 {"7"=TRUE, "6"=TRUE, "5"=TRUE, "4"=TRUE, "3"=TRUE, "2"=TRUE, "1"=TRUE} ("簇") T2 {"7"=TRUE, "6"=TRUE, "5"=TRUE, "4"=TRUE, "3"=FALSE, "2"=TRUE, "1"=TRUE} ("簇")] -> w273
          frame 0, Default {
          }
          frame 1 {
          }
          frame 2 {
          }
          frame 3 {
          }
          frame 4 {
          }
          frame 5 {
          }
          frame 6 {
          }
          frame 7 {
          }
          frame 8 {
          }
          frame 9 {
          }
        }
        "蓝方胜场比分十位" <- w273
      }
      frame 15 {
        n493 = Quotient & Remainder(x=w297, y=10) -> (x-y*floor(x/y)=w294:i32, floor(x/y)=w295:i32)
        n494 = case shown="1" w294 {
          tunnel: [T2 {"7"=TRUE, "6"=TRUE, "5"=TRUE, "4"=TRUE, "3"=TRUE, "2"=TRUE, "1"=FALSE} ("簇") T2 {"7"=FALSE, "6"=TRUE, "5"=TRUE, "4"=FALSE, "3"=FALSE, "2"=FALSE, "1"=FALSE} ("簇") T2 {"7"=TRUE, "6"=TRUE, "5"=FALSE, "4"=TRUE, "3"=TRUE, "2"=FALSE, "1"=TRUE} ("簇") T2 {"7"=TRUE, "6"=TRUE, "5"=TRUE, "4"=TRUE, "3"=FALSE, "2"=FALSE, "1"=TRUE} ("簇") T2 {"7"=FALSE, "6"=TRUE, "5"=TRUE, "4"=FALSE, "3"=FALSE, "2"=TRUE, "1"=TRUE} ("簇") T2 {"7"=TRUE, "6"=FALSE, "5"=TRUE, "4"=TRUE, "3"=FALSE, "2"=TRUE, "1"=TRUE} ("簇") T2 {"7"=TRUE, "6"=FALSE, "5"=TRUE, "4"=TRUE, "3"=TRUE, "2"=TRUE, "1"=TRUE} ("簇") T2 {"7"=TRUE, "6"=TRUE, "5"=TRUE, "4"=FALSE, "3"=FALSE, "2"=FALSE, "1"=FALSE} ("簇") T2 {"7"=TRUE, "6"=TRUE, "5"=TRUE, "4"=TRUE, "3"=TRUE, "2"=TRUE, "1"=TRUE} ("簇") T2 {"7"=TRUE, "6"=TRUE, "5"=TRUE, "4"=TRUE, "3"=FALSE, "2"=TRUE, "1"=TRUE} ("簇")] -> w296
          frame 0, Default {
          }
          frame 1 {
          }
          frame 2 {
          }
          frame 3 {
          }
          frame 4 {
          }
          frame 5 {
          }
          frame 6 {
          }
          frame 7 {
          }
          frame 8 {
          }
          frame 9 {
          }
        }
        "比赛次数个位" <- w296
        n495 = case shown="1" w295 {
          tunnel: [T2 {"7"=TRUE, "6"=TRUE, "5"=TRUE, "4"=TRUE, "3"=TRUE, "2"=TRUE, "1"=FALSE} ("簇") T2 {"7"=FALSE, "6"=TRUE, "5"=TRUE, "4"=FALSE, "3"=FALSE, "2"=FALSE, "1"=FALSE} ("簇") T2 {"7"=TRUE, "6"=TRUE, "5"=FALSE, "4"=TRUE, "3"=TRUE, "2"=FALSE, "1"=TRUE} ("簇") T2 {"7"=TRUE, "6"=TRUE, "5"=TRUE, "4"=TRUE, "3"=FALSE, "2"=FALSE, "1"=TRUE} ("簇") T2 {"7"=FALSE, "6"=TRUE, "5"=TRUE, "4"=FALSE, "3"=FALSE, "2"=TRUE, "1"=TRUE} ("簇") T2 {"7"=TRUE, "6"=FALSE, "5"=TRUE, "4"=TRUE, "3"=FALSE, "2"=TRUE, "1"=TRUE} ("簇") T2 {"7"=TRUE, "6"=FALSE, "5"=TRUE, "4"=TRUE, "3"=TRUE, "2"=TRUE, "1"=TRUE} ("簇") T2 {"7"=TRUE, "6"=TRUE, "5"=TRUE, "4"=FALSE, "3"=FALSE, "2"=FALSE, "1"=FALSE} ("簇") T2 {"7"=TRUE, "6"=TRUE, "5"=TRUE, "4"=TRUE, "3"=TRUE, "2"=TRUE, "1"=TRUE} ("簇") T2 {"7"=TRUE, "6"=TRUE, "5"=TRUE, "4"=TRUE, "3"=FALSE, "2"=TRUE, "1"=TRUE} ("簇")] -> w299
          frame 0, Default {
          }
          frame 1 {
          }
          frame 2 {
          }
          frame 3 {
          }
          frame 4 {
          }
          frame 5 {
          }
          frame 6 {
          }
          frame 7 {
          }
          frame 8 {
          }
          frame 9 {
          }
        }
        "比赛次数十位" <- w299
      }
      frame 16 {
        n496 = case shown="2" w321 {
          tunnel: [cluster{u32, u32}[] [{12369084, 16448250}] ("颜色[4]") cluster{u32, u32}[] [{12369084, 65379}] ("颜色[4]") cluster{u32, u32}[] [{12369084, 16776002}] ("颜色[4]") cluster{u32, u32}[] [{12369084, 16715776}] ("颜色[4]")] -> w320
          frame 0, 1, Default {
          }
          frame 2 {
          }
          frame 3 {
          }
          frame 4 {
          }
        }
        n497 = property on="比赛状态" class="Bool (严格)"("Colors [4]"=w320) -> ()  [unwired: 2 in, 2 out]
      }
    }
  }
  n498 = while {
    tunnel: [w335] -> w13
    tunnel: [w334] -> w12
    tunnel: w6 -> [w333]
    tunnel: w5 -> [w332]
    tunnel: w2 -> [w329]
    tunnel: [w329] -> w1
    stop <- "停止" stop-if-true
    n499 = case shown="True" "?" {
      tunnel: w333 -> [w419 w424]
      tunnel: w332 -> [w420 w425]
      tunnel: [w420 w422] -> w343
      tunnel: [w419 w421] -> w342
      frame False {
      }
      frame True {
        n500 = Byte Array To String(unsigned byte array=u8[] [17]) -> (string=w423:string)
        n501 = VISA Write(VISA resource name=w424, write buffer=w423, error in (no error)=w425) -> (VISA resource name out=w421:refnum<visa-resource-name>, error out=w422:errorcluster)  [unwired: 1 out]
      }
    }
    n502 = case shown="True" "?" {
      tunnel: w342 -> [w412 w416]
      tunnel: w343 -> [w411 w415]
      tunnel: [w412 w414] -> w341
      tunnel: [w411 w413] -> w340
      frame False {
      }
      frame True {
        n503 = Byte Array To String(unsigned byte array=u8[] [18] ("无符号字节数组")) -> (string=w417:string)
        n504 = VISA Write(VISA resource name=w416, write buffer=w417, error in (no error)=w415) -> (VISA resource name out=w414:refnum<visa-resource-name>, error out=w413:errorcluster)  [unwired: 1 out]
      }
    }
    n505 = case shown="True" "?" {
      tunnel: w341 -> [w404 w408]
      tunnel: w340 -> [w403 w407]
      tunnel: [w404 w406] -> w347
      tunnel: [w403 w405] -> w346
      frame False {
      }
      frame True {
        n506 = Byte Array To String(unsigned byte array=u8[] [19] ("无符号字节数组")) -> (string=w409:string)
        n507 = VISA Write(VISA resource name=w408, write buffer=w409, error in (no error)=w407) -> (VISA resource name out=w406:refnum<visa-resource-name>, error out=w405:errorcluster)  [unwired: 1 out]
      }
    }
    n508 = property class="Instr"(reference=w347, error in=w346) -> (reference out=w338:refnum<visa-resource-name>, error out=w337:errorcluster, "Serial Settings:Number of Bytes at Serial Port"=w339:u32)
    "Number of Bytes" <- w339
    n509 = Greater Than 0?(x=w339) -> (x > 0?=w336:bool)
    n510 = case shown="True" w336 {
      tunnel: [0 w384] -> w330
      tunnel: [u8 0 w383] -> w327
      tunnel: [w376 w381] -> w335
      tunnel: [w375 w380] -> w334
      tunnel: w338 -> [w375 w379]
      tunnel: w337 -> [w376 w377]
      frame False {
      }
      frame True {
        n511 = VISA Read(VISA resource name=w379, byte count=u32 1 ("字节总数"), error in (no error)=w377) -> (VISA resource name out=w382:refnum<visa-resource-name>, read buffer=w388:string, error out=w378:errorcluster)  [unwired: 1 out]
        "读取缓冲区 5" <- w388
        n512 = String To Byte Array(string=w388) -> (unsigned byte array=w387:u8[])
        n513 = Index Array(array=w387, index=0 ("索引")) -> (element=w383:u8)
        n514 = case shown="2, 10..13, 15, 16" w383 {
          tunnel: [w393 0] -> w384
          tunnel: w382 -> [w392 w402]
          tunnel: w378 -> [w391 w401]
          tunnel: [w390 w401] -> w381
          tunnel: [w389 w402] -> w380
          frame 2, 10..13, 15, 16 {
            n515 = VISA Read(VISA resource name=w392, byte count=4 ("索引"), error in (no error)=w391) -> (VISA resource name out=w389:refnum<visa-resource-name>, read buffer=w397:string, error out=w398:errorcluster)  [unwired: 1 out]
            n516 = Unflatten From String(type=0, binary string=w397, data includes array or string size? (T)=FALSE ("数据中包含数组或字符串大小？(T)"), byte order (0:big-endian, network order)=T3."native, host order" ("字节顺序(0:big-endian, network order)"), error in (no error)=w398) -> (value=w393:i32, error out=w390:errorcluster)  [unwired: 1 out]
          }
          frame Default {
          }
        }
      }
    }
    n517 = Greater Than 0?(x=w327) -> (x > 0?=w326:bool)
    n518 = case shown="True" w326 {
      tunnel: w327 -> [_ w348]
      tunnel: w330 -> [_ w351]
      tunnel: w329 -> [_ w349]
      frame False {
      }
      frame True {
        n519 = Equal?(x=w348, y=u8 16) -> (x = y?=w353:bool)
        n520 = Equal?(x=w351, y=u8 2) -> (x = y?=w352:bool)
        n521 = And(x=w353, y=w352) -> (x .and. y?=w354:bool)
        n522 = case shown="True" w354 {
          tunnel: w351 -> [w359 w361]
          tunnel: w349 -> [w357 w360]
          tunnel: w348 -> [w356 _]
          frame False {
            n523 = Build Array(w356, w359) -> (w358:i32[])
            n524 = Enqueue Element(queue=w357, element=w358) -> ()  [unwired: 2 in, 3 out]
          }
          frame True {
            w362 = i32[] [11, 10, 16]
            n525 = Array Size(array=w362) -> (size(s)=w363:i32)
            n526 = for {
              N: w363 -> [_]
              tunnel: w362 -> [w364] mode=indexing
              tunnel: w361 -> [w368]
              tunnel: w360 -> [w366]
              n527 = Equal?(x=w364, y=16 ("x")) -> (x = y?=w369:bool)
              n528 = case shown="False" w369 {
                tunnel: w368 -> [_ w372]
                tunnel: [0 w372] -> w367
                frame False {
                }
                frame True {
                }
              }
              n529 = Build Array(w364, w367) -> (w365:i32[])
              n530 = Enqueue Element(queue=w366, element=w365) -> ()  [unwired: 2 in, 3 out]
            }
          }
        }
      }
    }
  }
  n531 = property on="候场/暂停" class="Bool (严格)"("Colors [4]"=cluster{u32, u32}[] [{12369084, 16776002}] ("颜色[4]")) -> ()  [unwired: 2 in, 2 out]
  n532 = property on="结束" class="Bool (严格)"("Colors [4]"=cluster{u32, u32}[] [{12369084, 16711680}] ("颜色[4]")) -> ()  [unwired: 2 in, 2 out]
  n533 = VISA Close(VISA resource name=w12, error in (no error)=w13) -> (error out=w14:errorcluster)
  n534 = Release Queue(queue=w1) -> ()  [unwired: 2 in, 3 out]
  n535 = call <vilib>:"Simple Error Handler.vi"("error in (no error)"=w14) -> ()  [unwired: 4 in, 5 out]
  "指示灯2" <- w16
  "指示灯1" <- w16
  "指示灯2 2" <- w15
  "指示灯1 2" <- w15
  "计时" <- TRUE
